vi "Wago DO Arrange.vi"(0 "Wago Data Input in":T2 {"Input Process Image"."Software Constants"."Room PID Settings"."Room Dehumid Temperature I (*RM Dehum I1)" max=30000 step=1; "Input Process Image"."Software Constants"."Room PID Settings"."Room Dehumid Temperature P (*RM Dehum P1)" max=30000 step=1; "Input Process Image"."Software Constants"."Room PID Settings"."Room Cool Temperature I (*RM Cool I1)" max=30000 step=1; "Input Process Image"."Software Constants"."Room PID Settings"."Room Cool Temperature P (*RM Cool P1)" max=30000 step=1; "Input Process Image"."Software Constants"."Room PID Settings"."Room Heat I (*RM Heat I1)" max=30000 step=1; "Input Process Image"."Software Constants"."Room PID Settings"."Room Heat P (*RM Heat P1)" max=30000 step=1; "Input Process Image"."Software Constants"."Room PID Settings"."Room Humidity I (*RM Hum I1)" max=30000 step=1; "Input Process Image"."Software Constants"."Room PID Settings"."Room Humidity P (*RM Hum P1)" max=30000 step=1; "Input Process Image"."Software Constants"."Room PID Settings"."Room Dry I (*RM Dry I1)" max=30000 step=1; "Input Process Image"."Software Constants"."Room PID Settings"."Room Dry P(*RM Dry P1)" max=30000 step=1}, 5 "Flipped Bytes (16 bits)":bool[](array[boolean]), 11 "Error In":errorcluster, 12 "Wago Output Words":T1=519 items=["twHeatCtrl"=512, "twSteamCtrl"=513, "twCoolCtrl"=514, "twDehumCtrl"=515, "Output QX4 Bool"=516, "Output QX5 Bool"=517, "Output QX6 Bool"=518, "Output QX7 Bool"=519, "Output QX8 Bool"=520, "Output QX9 Bool"=521, "Output QX10"=522, "twRoomTemp"=840, "twRoomHum"=841, "twSuppTemp"=842, "twCoolTemp"=843, "twDehumTemp"=844, "twGlycolTemp"=845, "twHeatRate"=846, "twSteamRate"=847, "twCoolRate"=848, "twDehumRate"=849, "twStatus"=850, "twDoorEna"=851, "Rm1St1Dr1Stat"=816, "Rm1St2Dr1Stat"=817, "Rm1St3Dr1Stat"=818, "Rm1St4Dr1Stat"=819, "Rm1St5Dr1Stat"=820, "Rm1St6Dr1Stat"=821, "Rm1St7Dr1Stat"=822, "Rm1St8Dr1Stat"=823, "Rm1St1Dr2Stat"=824, "Rm1St2Dr2Stat"=825, "Rm1St3Dr2Stat"=826, "Rm1St4Dr2Stat"=827, "Rm1St5Dr2Stat"=828, "Rm1St6DrStat"=829, "Rm1St7Dr2Stat"=830, "Rm1St8Dr2Stat"=831, "Rm1St1Dr3Stat"=832, "Rm1St2Dr3Stat"=833, "Rm1St3Dr3Stat"=834, "Rm1St4Dr3Stat"=835, "Rm1St5Dr3Stat"=836, "Rm1St6Dr3Stat"=837, "Rm1St7Dr3Stat"=838, "Rm1St8Dr3Stat"=839, "twVoltMon1"=784, "twVoltMon2"=785, "twVoltMon3"=786, "twVoltMon4"=787, "twVoltMon5"=788, "twVoltMon6"=789, "twVoltMon7"=790, "twVoltMon8"=791, "twVoltStat1"=792, "twVoltStat2"=793, "twVoltStat3"=794, "twVoltStat4"=795, "twVoltStat5"=796, "twVoltStat6"=797, "twVoltStat7"=798, "twVoltStat8"=799]) -> (4 "Wago Data Input out":T2 {"Input Process Image"."Software Constants"."Room PID Settings"."Room Dehumid Temperature I (*RM Dehum I1)" max=30000 step=1; "Input Process Image"."Software Constants"."Room PID Settings"."Room Dehumid Temperature P (*RM Dehum P1)" max=30000 step=1; "Input Process Image"."Software Constants"."Room PID Settings"."Room Cool Temperature I (*RM Cool I1)" max=30000 step=1; "Input Process Image"."Software Constants"."Room PID Settings"."Room Cool Temperature P (*RM Cool P1)" max=30000 step=1; "Input Process Image"."Software Constants"."Room PID Settings"."Room Heat I (*RM Heat I1)" max=30000 step=1; "Input Process Image"."Software Constants"."Room PID Settings"."Room Heat P (*RM Heat P1)" max=30000 step=1; "Input Process Image"."Software Constants"."Room PID Settings"."Room Humidity I (*RM Hum I1)" max=30000 step=1; "Input Process Image"."Software Constants"."Room PID Settings"."Room Humidity P (*RM Hum P1)" max=30000 step=1; "Input Process Image"."Software Constants"."Room PID Settings"."Room Dry I (*RM Dry I1)" max=30000 step=1; "Input Process Image"."Software Constants"."Room PID Settings"."Room Dry P(*RM Dry P1)" max=30000 step=1}, 15 "Error Out":errorcluster)   [LabVIEW 2016]
uses:
  Type Definitions/Wago Main Control.ctl
  Type Definitions/Wago Output Data Process Image.ctl
  Type Definitions/Wago Room Condtions.ctl
  Type Definitions/Wago Door Relays.ctl
  Type Definitions/Wago Contactor Settings.ctl
  Type Definitions/Wago Ground Leakage.ctl
  Type Definitions/Wago Input Process Image.ctl
  Type Definitions/Wago Room PID Settings.ctl
  Type Definitions/Wago Measured Input Data.ctl
  Type Definitions/Wago Room Setpoint Targets.ctl
  Type Definitions/Wago Output Commands.ctl
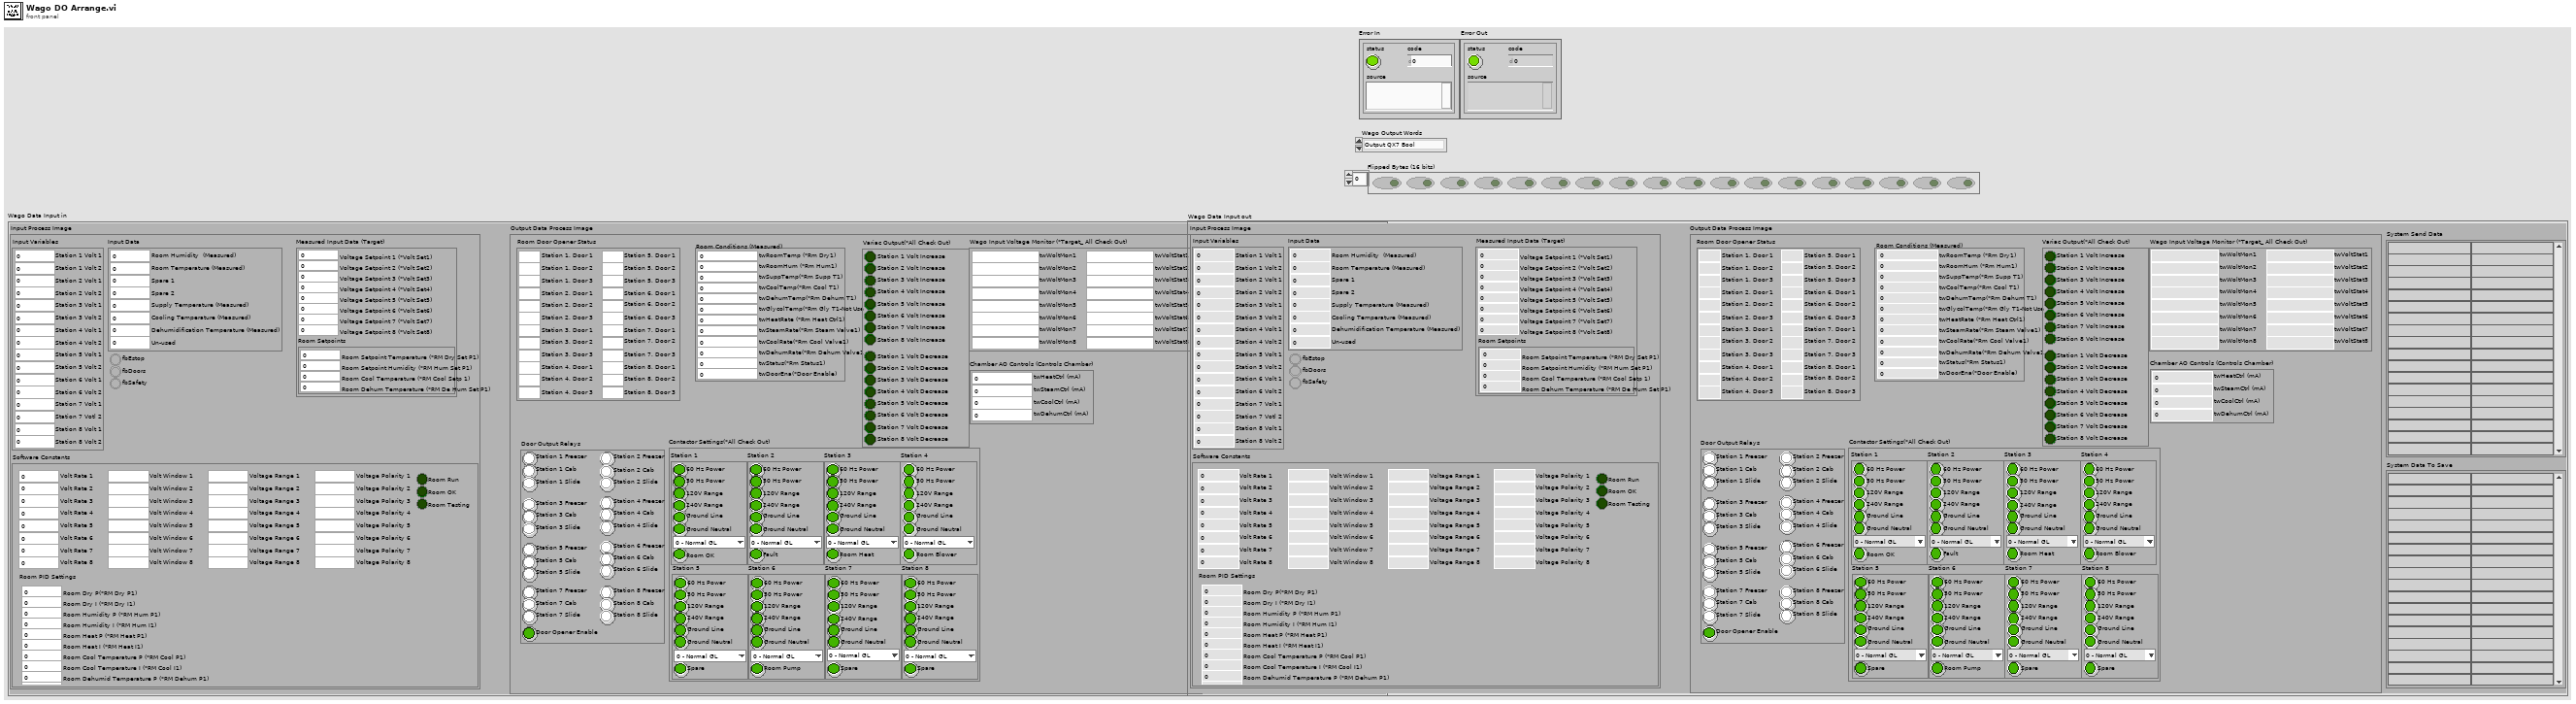
[diagram p1: front panel]
types:
  T1 = typedef "Wago Output Commands.ctl" = u16
  T2 = typedef "Wago Main Control.ctl" = cluster{"Output Data Process Image":T3, "Input Process Image":T8, "System Send Data":string[][], "System Data To Save":string[][]}
  T3 = typedef "Wago Output Data Process Image.ctl" = cluster{"Room Door Opener Status":cluster{"Station 1, Door 1":u16, "Station 1, Door 2":u16, "Station 1, Door 3":u16, "Station 2, Door 1":u16, "Station 2, Door 2":u16, "Station 2, Door 3":u16, "Station 3, Door 1":u16, "Station 3, Door 2":u16, "Station 3, Door 3":u16, "Station 4, Door 1":u16, "Station 4, Door 2":u16, "Station 4, Door 3":u16, "Station 5, Door 1":u16, "Station 5, Door 2":u16, "Station 5, Door 3":u16, "Station 6, Door 1":u16, "Station 6, Door 2":u16, "Station 6, Door 3":u16, "Station 7, Door 1":u16, "Station 7, Door 2":u16, "Station 7, Door 3":u16, "Station 8, Door 1":u16, "Station 8, Door 2":u16, "Station 8, Door 3":u16}, "Room Conditions (Measured)":T4, "Chamber AO Controls (Controls Chamber)":cluster{"twDehumCtrl (mA)":u16, "twCoolCtrl (mA)":u16, "twSteamCtrl (mA)":u16, "twHeatCtrl (mA)":u16}, "Variac Output(*All Check Out)":cluster{"Station 1 Volt Increase":bool, "Station 1 Volt Decrease":bool, "Station 2 Volt Increase":bool, "Station 2 Volt Decrease":bool, "Station 3 Volt Increase":bool, "Station 3 Volt Decrease":bool, "Station 4 Volt Increase":bool, "Station 4 Volt Decrease":bool, "Station 5 Volt Increase":bool, "Station 5 Volt Decrease":bool, "Station 6 Volt Increase":bool, "Station 6 Volt Decrease":bool, "Station 7 Volt Increase":bool, "Station 7 Volt Decrease":bool, "Station 8 Volt Increase":bool, "Station 8 Volt Decrease":bool}, "Door Output Relays":T5, "Wago Input Voltage Monitor (*Target_ All Check Out)":cluster{"twWoltMon1":dbl, "twWoltMon2":dbl, "twWoltMon3":dbl, "twWoltMon4":dbl, "twWoltMon5":dbl, "twWoltMon6":dbl, "twWoltMon7":dbl, "twWoltMon8":dbl, "twVoltStat1":u16, "twVoltStat2":u16, "twVoltStat3":u16, "twVoltStat4":u16, "twVoltStat5":u16, "twVoltStat6":u16, "twVoltStat7":u16, "twVoltStat8":u16}, "Contactor Settings(*All Check Out)":T6}
  T4 = typedef "Wago Room Condtions.ctl" = cluster{"twDoorEna(*Door Enable)":u16, "twStatus(*Rm Status1)":u16, "twRoomTemp (*Rm Dry1)":dbl, "twRoomHum (*Rm Hum1)":dbl, "twSuppTemp(*Rm Supp T1)":dbl, "twCoolTemp(*Rm Cool T1)":dbl, "twDehumTemp(*Rm Dehum T1)":dbl, "twGlycolTemp(*Rm Gly T1-Not Used)":dbl, "twDehumRate(*Rm Dehum Valve1)":dbl, "twCoolRate(*Rm Cool Valve1)":dbl, "twSteamRate(*Rm Steam Valve1)":dbl, "twHeatRate (*Rm Heat Ctrl1)":dbl}
  T5 = typedef "Wago Door Relays.ctl" = cluster{"Station 1 Freezer":bool, "Station 1 Cab":bool, "Station 1 Slide":bool, "Station 2 Freezer":bool, "Station 2 Cab":bool, "Station 2 Slide":bool, "Station 3 Freezer":bool, "Station 3 Cab":bool, "Station 3 Slide":bool, "Station 4 Freezer":bool, "Station 4 Cab":bool, "Station 4 Slide":bool, "Station 5 Freezer":bool, "Station 5 Cab":bool, "Station 5 Slide":bool, "Station 6 Freezer":bool, "Station 6 Cab":bool, "Station 6 Slide":bool, "Station 7 Freezer":bool, "Station 7 Cab":bool, "Station 7 Slide":bool, "Station 8 Freezer":bool, "Station 8 Cab":bool, "Station 8 Slide":bool, "Door Opener Enable":bool}
  T6 = typedef "Wago Contactor Settings.ctl" = cluster{"Station 1":cluster{"60 Hz Power":bool, "50 Hz Power":bool, "120V Range":bool, "240V Range":bool, "Ground Line":bool, "Ground Neutral":bool, "Room OK":bool, "Ground Leakage":T7}, "Station 2":cluster{"60 Hz Power":bool, "50 Hz Power":bool, "120V Range":bool, "240V Range":bool, "Ground Line":bool, "Ground Neutral":bool, "Fault":bool, "Ground Leakage":T7}, "Station 3":cluster{"60 Hz Power":bool, "50 Hz Power":bool, "120V Range":bool, "240V Range":bool, "Ground Line":bool, "Ground Neutral":bool, "Room Heat":bool, "Ground Leakage":T7}, "Station 4":cluster{"60 Hz Power":bool, "50 Hz Power":bool, "120V Range":bool, "240V Range":bool, "Ground Line":bool, "Ground Neutral":bool, "Room Blower":bool, "Ground Leakage":T7}, "Station 5":cluster{"60 Hz Power":bool, "50 Hz Power":bool, "120V Range":bool, "240V Range":bool, "Ground Line":bool, "Ground Neutral":bool, "Spare":bool, "Ground Leakage":T7}, "Station 6":cluster{"60 Hz Power":bool, "50 Hz Power":bool, "120V Range":bool, "240V Range":bool, "Ground Line":bool, "Ground Neutral":bool, "Room Pump":bool, "Ground Leakage":T7}, "Station 7":cluster{"60 Hz Power":bool, "50 Hz Power":bool, "120V Range":bool, "240V Range":bool, "Ground Line":bool, "Ground Neutral":bool, "Spare":bool, "Ground Leakage":T7}, "Station 8":cluster{"60 Hz Power":bool, "50 Hz Power":bool, "120V Range":bool, "240V Range":bool, "Ground Line":bool, "Ground Neutral":bool, "Spare":bool, "Ground Leakage":T7}}
  T7 = typedef "Wago Ground Leakage.ctl" = enum16{"0 - Normal GL", "1 - Measure GL"}
  T8 = typedef "Wago Input Process Image.ctl" = cluster{"fbEstop":bool, "fbDoors":bool, "fbSafety":bool, "Input Variables":cluster{"Station 1 Volt 1":dbl, "Station 1 Volt 2":dbl, "Station 2 Volt 1":dbl, "Station 2 Volt 2":dbl, "Station 3 Volt 1":dbl, "Station 3 Volt 2":dbl, "Station 4 Volt 1":dbl, "Station 4 Volt 2":dbl, "Station 5 Volt 1":dbl, "Station 5 Volt 2":dbl, "Station 6 Volt 1":dbl, "Station 6 Volt 2":dbl, "Station 7 Volt 1":dbl, "Station 7 Votl 2":dbl, "Station 8 Volt 1":dbl, "Station 8 Volt 2":dbl}, "Input Data":cluster{"Room Humidity  (Measured)":dbl, "Room Temperature (Measured)":dbl, "Spare 1":dbl, "Spare 2":dbl, "Supply Temperature (Measured)":dbl, "Cooling Temperature (Measured)":dbl, "Dehumidification Temperature (Measured)":dbl, "Un-used":dbl}, "Software Constants":cluster{"Volt Rate 1":u16, "Volt Rate 2":u16, "Volt Rate 3":u16, "Volt Rate 4":u16, "Volt Rate 5":u16, "Volt Rate 6":u16, "Volt Rate 7":u16, "Volt Rate 8":u16, "Volt Window 1":u16, "Volt Window 2":u16, "Volt Window 3":u16, "Volt Window 4":u16, "Volt Window 5":u16, "Volt Window 6":u16, "Volt Window 7":u16, "Volt Window 8":u16, "Voltage Range 1":u16, "Voltage Range 2":u16, "Voltage Range 3":u16, "Voltage Range 4":u16, "Voltage Range 5":u16, "Voltage Range 6":u16, "Voltage Range 7":u16, "Voltage Range 8":u16, "Voltage Polarity 1":u16, "Voltage Polarity 2":u16, "Voltage Polarity 3":u16, "Voltage Polarity 4":u16, "Voltage Polarity 5":u16, "Voltage Polarity 6":u16, "Voltage Polarity 7":u16, "Voltage Polarity 8":u16, "Room Run":bool, "Room OK":bool, "Room Testing":bool, "Room PID Settings":T9}, "Measured Input Data (Target)":T10}
  T9 = typedef "Wago Room PID Settings.ctl" = cluster{"Room Dry P(*RM Dry P1)":u16, "Room Dry I (*RM Dry I1)":u16, "Room Humidity P (*RM Hum P1)":u16, "Room Humidity I (*RM Hum I1)":u16, "Room Heat P (*RM Heat P1)":u16, "Room Heat I (*RM Heat I1)":u16, "Room Cool Temperature P (*RM Cool P1)":u16, "Room Cool Temperature I (*RM Cool I1)":u16, "Room Dehumid Temperature P (*RM Dehum P1)":u16, "Room Dehumid Temperature I (*RM Dehum I1)":u16}
  T10 = typedef "Wago Measured Input Data.ctl" = cluster{"Voltage Setpoint 1 (*Volt Set1)":dbl, "Voltage Setpoint 2 (*Volt Set2)":dbl, "Voltage Setpoint 3 (*Volt Set3)":dbl, "Voltage Setpoint 4 (*Volt Set4)":dbl, "Voltage Setpoint 5 (*Volt Set5)":dbl, "Voltage Setpoint 6 (*Volt Set6)":dbl, "Voltage Setpoint 7 (*Volt Set7)":dbl, "Voltage Setpoint 8 (*Volt Set8)":dbl, "Room Setpoints":T11}
  T11 = typedef "Wago Room Setpoint Targets.ctl" = cluster{"Room Setpoint Temperature (*RM Dry Set P1)":dbl, "Room Setpoint Humidity (*RM Hum Set P1)":dbl, "Room Cool Temperature (*RM Cool Setp 1)":dbl, "Room Dehum Temperature (*RM De Hum Set P1)":dbl}
  T12 = cluster{"60 Hz Power":bool, "50 Hz Power":bool, "120V Range":bool, "240V Range":bool, "Ground Line":bool, "Ground Neutral":bool, "Room OK":bool, "Ground Leakage":T7}
  T13 = cluster{"60 Hz Power":bool, "50 Hz Power":bool, "120V Range":bool, "240V Range":bool, "Ground Line":bool, "Ground Neutral":bool, "Fault":bool, "Ground Leakage":T7}
  T14 = cluster{"60 Hz Power":bool, "50 Hz Power":bool, "120V Range":bool, "240V Range":bool, "Ground Line":bool, "Ground Neutral":bool, "Room Heat":bool, "Ground Leakage":T7}
  T15 = cluster{"60 Hz Power":bool, "50 Hz Power":bool, "120V Range":bool, "240V Range":bool, "Ground Line":bool, "Ground Neutral":bool, "Room Blower":bool, "Ground Leakage":T7}
  T16 = cluster{"60 Hz Power":bool, "50 Hz Power":bool, "120V Range":bool, "240V Range":bool, "Ground Line":bool, "Ground Neutral":bool, "Spare":bool, "Ground Leakage":T7}
  T17 = cluster{"60 Hz Power":bool, "50 Hz Power":bool, "120V Range":bool, "240V Range":bool, "Ground Line":bool, "Ground Neutral":bool, "Room Pump":bool, "Ground Leakage":T7}
  T18 = cluster{"Station 1 Volt Increase":bool, "Station 1 Volt Decrease":bool, "Station 2 Volt Increase":bool, "Station 2 Volt Decrease":bool, "Station 3 Volt Increase":bool, "Station 3 Volt Decrease":bool, "Station 4 Volt Increase":bool, "Station 4 Volt Decrease":bool, "Station 5 Volt Increase":bool, "Station 5 Volt Decrease":bool, "Station 6 Volt Increase":bool, "Station 6 Volt Decrease":bool, "Station 7 Volt Increase":bool, "Station 7 Volt Decrease":bool, "Station 8 Volt Increase":bool, "Station 8 Volt Decrease":bool}
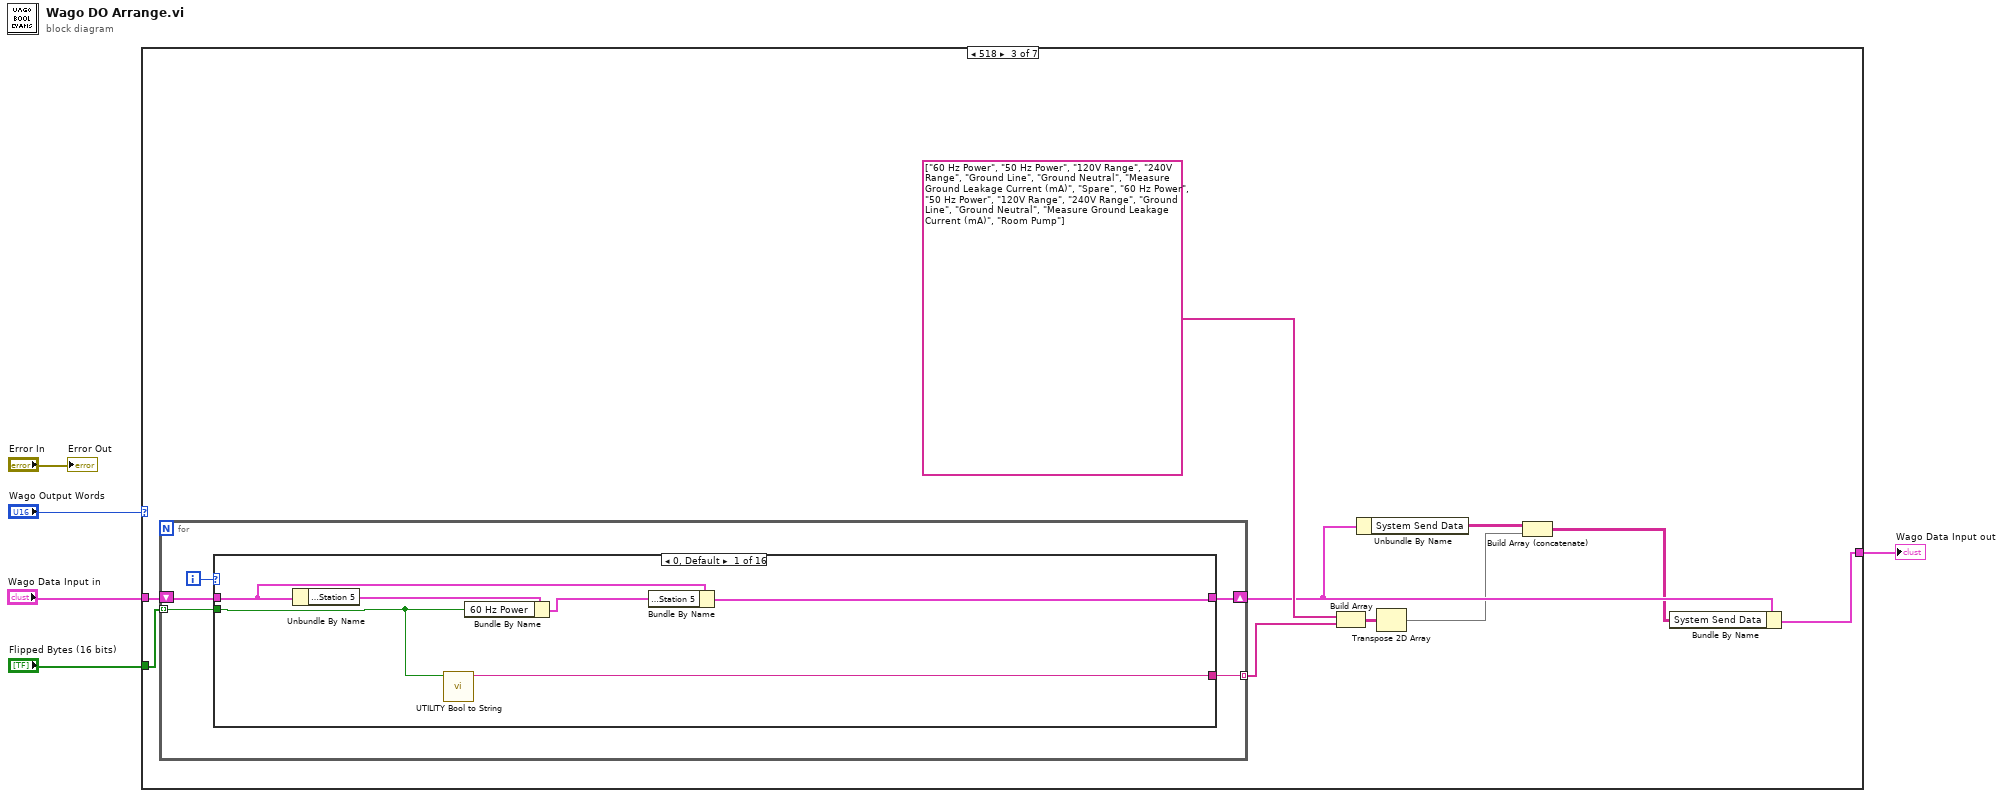
[diagram p0: block diagram]
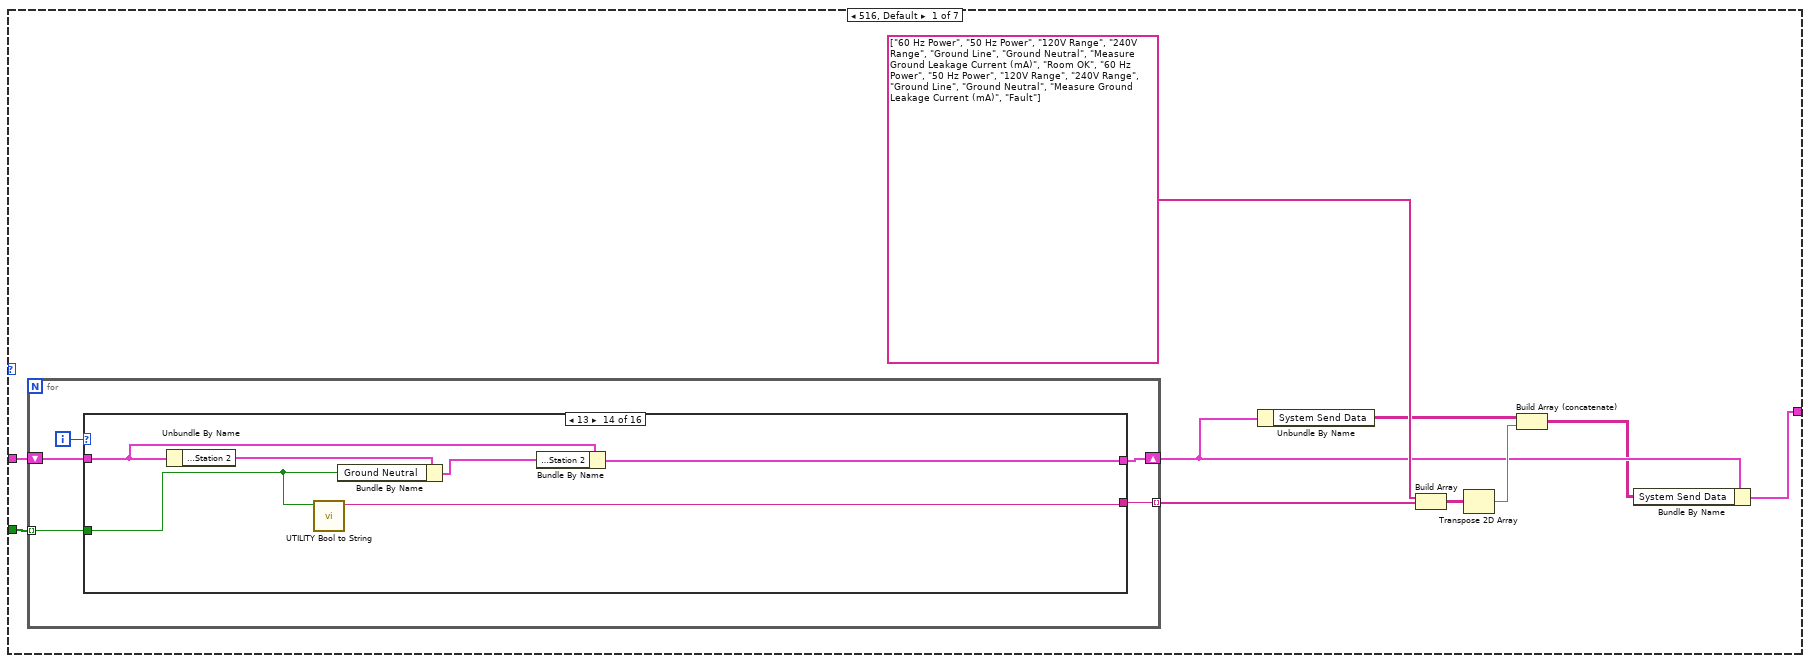
[diagram p2: hidden frame]
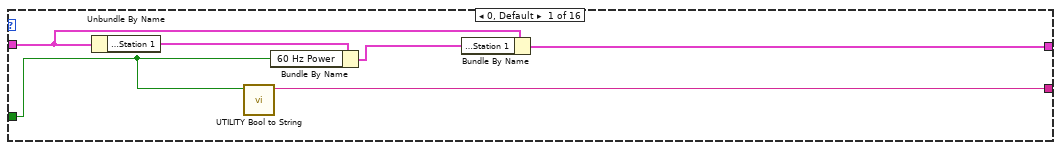
[diagram p3: hidden frame]
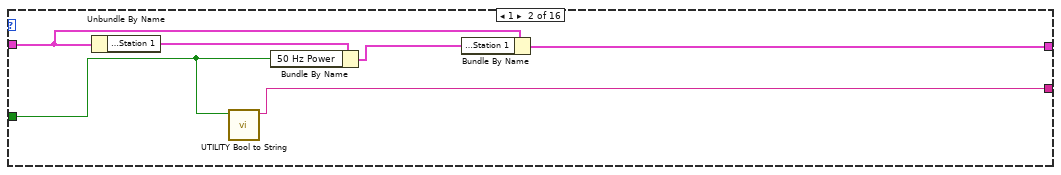
[diagram p4: hidden frame]
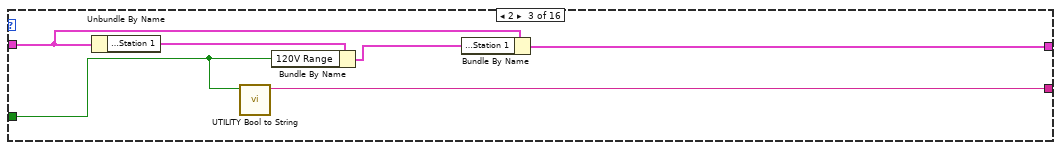
[diagram p5: hidden frame]
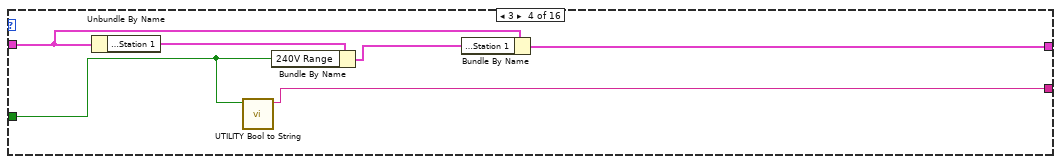
[diagram p6: hidden frame]
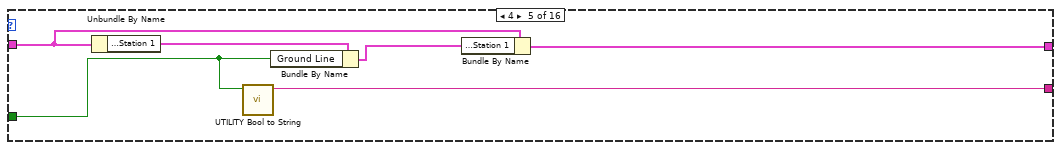
[diagram p7: hidden frame]
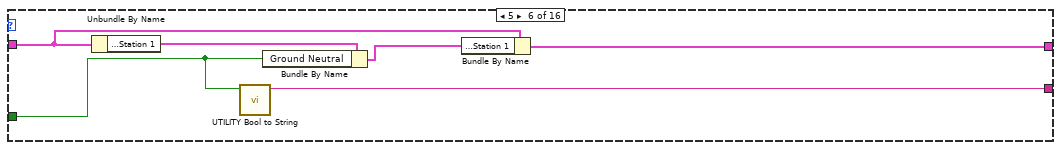
[diagram p8: hidden frame]
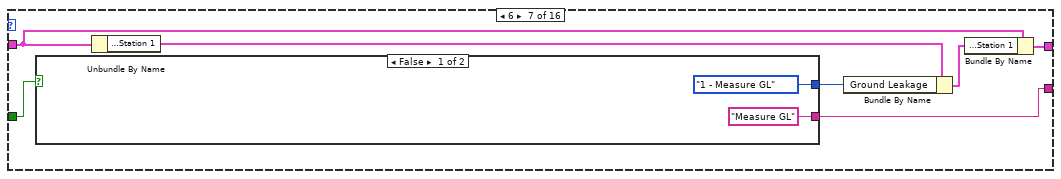
[diagram p9: hidden frame]
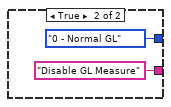
[diagram p10: hidden frame]
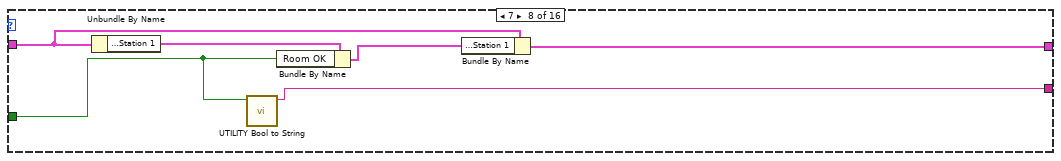
[diagram p11: hidden frame]
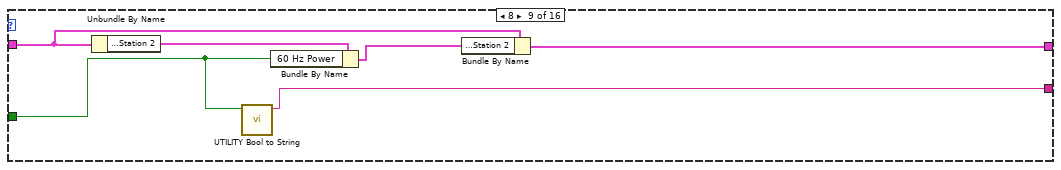
[diagram p12: hidden frame]
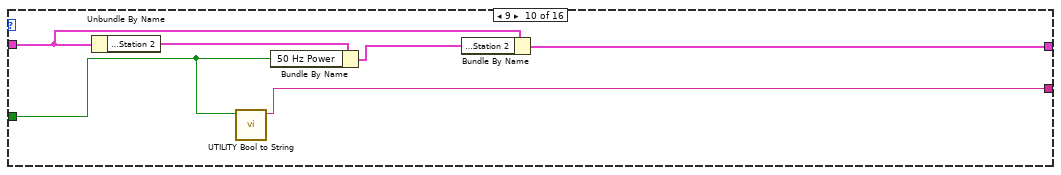
[diagram p13: hidden frame]
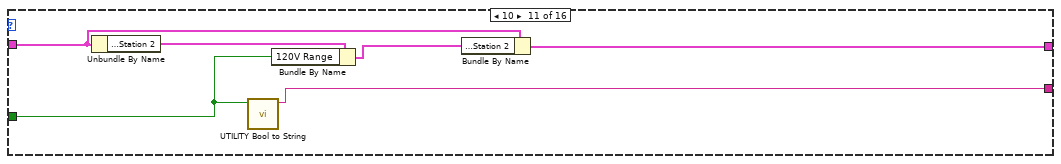
[diagram p14: hidden frame]
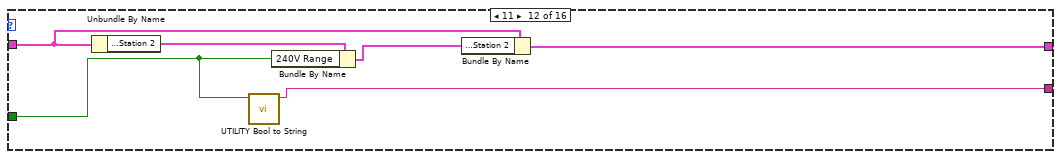
[diagram p15: hidden frame]
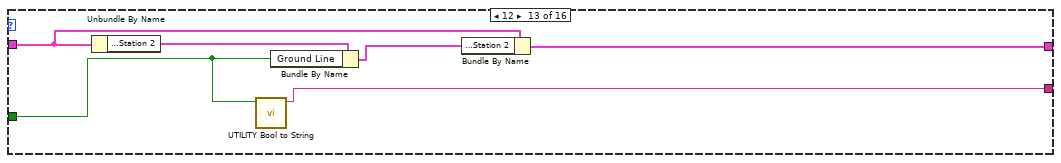
[diagram p16: hidden frame]
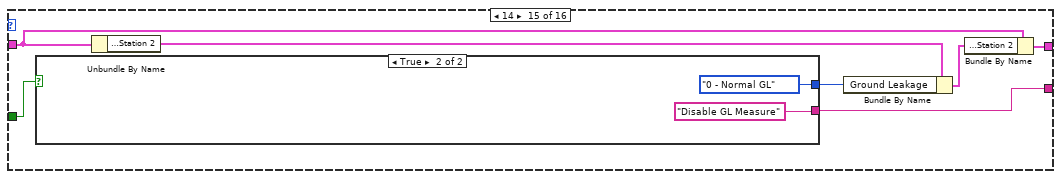
[diagram p17: hidden frame]
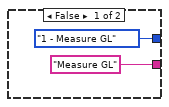
[diagram p18: hidden frame]
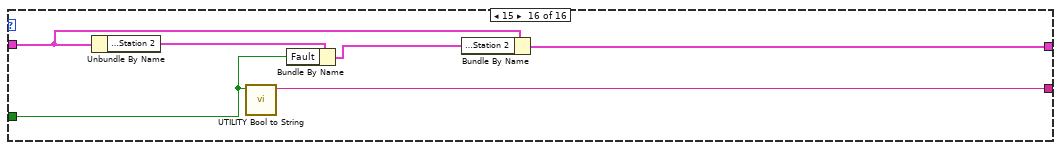
[diagram p19: hidden frame]
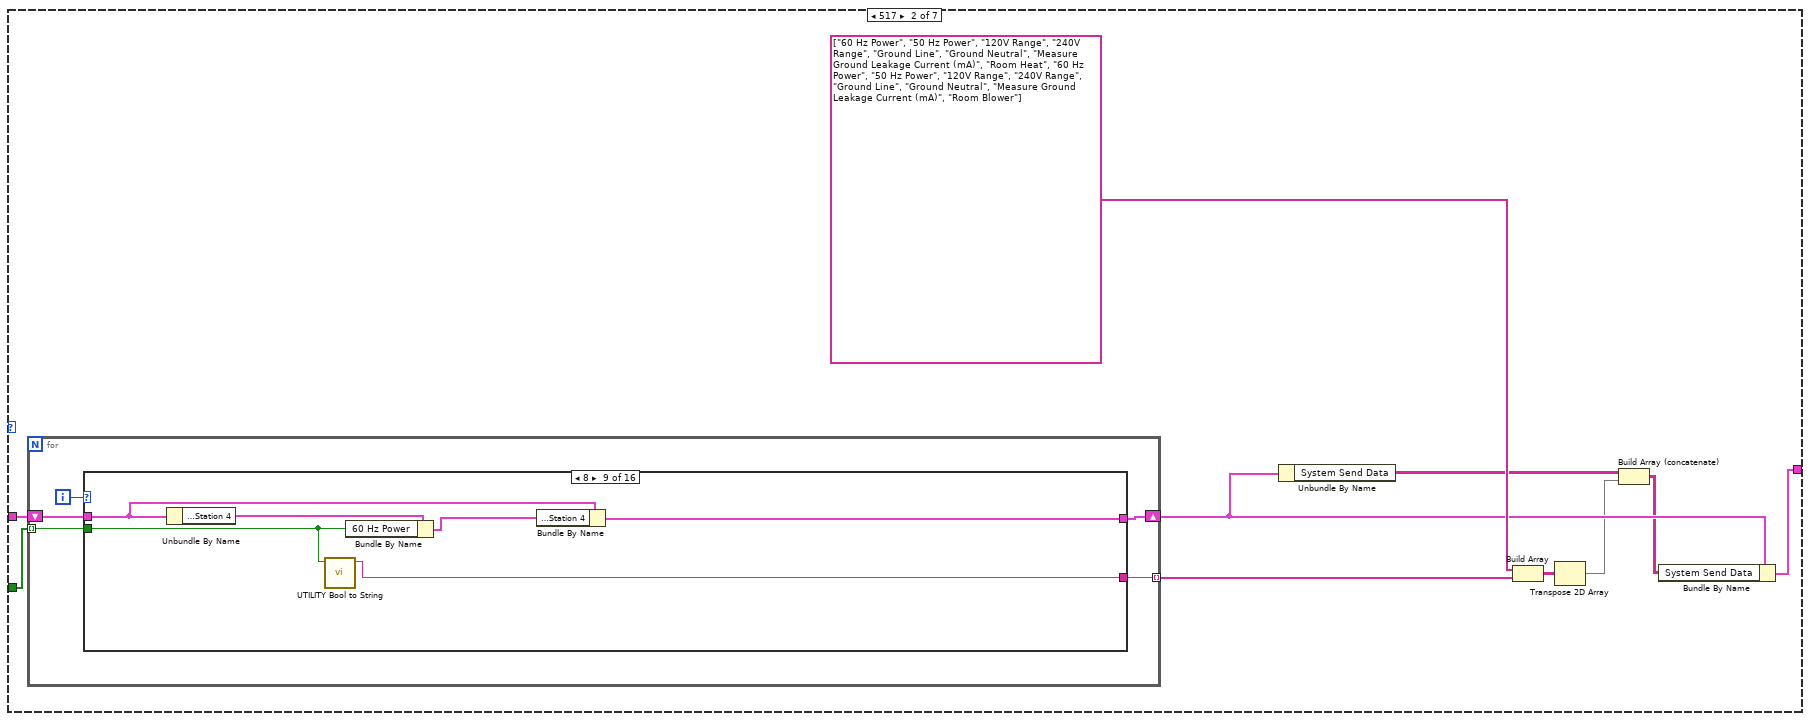
[diagram p20: hidden frame]
diagram:
  n1 = case shown="518" "Wago Output Words" {
    tunnel: "Wago Data Input in" -> [w15 w136 w257 w378 w499 w610 w722]
    tunnel: "Flipped Bytes (16 bits)" -> [w14 w135 w256 w377 w498 w609 w721]
    tunnel: [w10 w131 w254 w375 w496 w607 w718] -> w3
    frame 516, Default {
      n2 = for {
        tunnel: w14 -> [w18] mode=indexing
        shift-right: [w17] -> w8
        shift-left: w15 -> [w20]
        tunnel: [w16] -> w12 mode=indexing
        i -> [w19]
        n3 = case shown="13" w19 {
          tunnel: w20 -> [w25 w30 w36 w42 w48 w54 w61 w71 w77 w83 w89 w95 w101 w107 w114 w124]
          tunnel: w18 -> [w22 w28 w34 w40 w46 w52 w59 w69 w75 w81 w87 w93 w99 w105 w112 w122]
          tunnel: [w23 w29 w35 w41 w47 w53 w60 w70 w76 w82 w88 w94 w100 w106 w113 w123] -> w17
          tunnel: [w21 w27 w33 w39 w45 w51 w57 w68 w74 w80 w86 w92 w98 w104 w110 w121] -> w16
          frame 0, Default {
            n4 = Unbundle By Name(w25) -> ("Output Data Process Image.Contactor Settings(*All Check Out).Station 1"=w26:T12)
            n5 = call "UTILITY Bool to String.vi"("Input Bool"=w22) -> ("Output String"=w21:string)  [unwired: 10 in]
            n6 = Bundle By Name(cluster=w26, "60 Hz Power"=w22) -> (w24:T12)
            n7 = Bundle By Name(cluster=w25, "Output Data Process Image.Contactor Settings(*All Check Out).Station 1"=w24) -> (w23:T2)
          }
          frame 1 {
            n8 = Unbundle By Name(w30) -> ("Output Data Process Image.Contactor Settings(*All Check Out).Station 1"=w32:T12)
            n9 = call "UTILITY Bool to String.vi"("Input Bool"=w28) -> ("Output String"=w27:string)  [unwired: 10 in]
            n10 = Bundle By Name(cluster=w32, "50 Hz Power"=w28) -> (w31:T12)
            n11 = Bundle By Name(cluster=w30, "Output Data Process Image.Contactor Settings(*All Check Out).Station 1"=w31) -> (w29:T2)
          }
          frame 2 {
            n12 = Unbundle By Name(w36) -> ("Output Data Process Image.Contactor Settings(*All Check Out).Station 1"=w38:T12)
            n13 = call "UTILITY Bool to String.vi"("Input Bool"=w34) -> ("Output String"=w33:string)  [unwired: 10 in]
            n14 = Bundle By Name(cluster=w38, "120V Range"=w34) -> (w37:T12)
            n15 = Bundle By Name(cluster=w36, "Output Data Process Image.Contactor Settings(*All Check Out).Station 1"=w37) -> (w35:T2)
          }
          frame 3 {
            n16 = Unbundle By Name(w42) -> ("Output Data Process Image.Contactor Settings(*All Check Out).Station 1"=w44:T12)
            n17 = call "UTILITY Bool to String.vi"("Input Bool"=w40) -> ("Output String"=w39:string)  [unwired: 10 in]
            n18 = Bundle By Name(cluster=w44, "240V Range"=w40) -> (w43:T12)
            n19 = Bundle By Name(cluster=w42, "Output Data Process Image.Contactor Settings(*All Check Out).Station 1"=w43) -> (w41:T2)
          }
          frame 4 {
            n20 = Unbundle By Name(w48) -> ("Output Data Process Image.Contactor Settings(*All Check Out).Station 1"=w50:T12)
            n21 = call "UTILITY Bool to String.vi"("Input Bool"=w46) -> ("Output String"=w45:string)  [unwired: 10 in]
            n22 = Bundle By Name(cluster=w50, "Ground Line"=w46) -> (w49:T12)
            n23 = Bundle By Name(cluster=w48, "Output Data Process Image.Contactor Settings(*All Check Out).Station 1"=w49) -> (w47:T2)
          }
          frame 5 {
            n24 = Unbundle By Name(w54) -> ("Output Data Process Image.Contactor Settings(*All Check Out).Station 1"=w56:T12)
            n25 = call "UTILITY Bool to String.vi"("Input Bool"=w52) -> ("Output String"=w51:string)  [unwired: 10 in]
            n26 = Bundle By Name(cluster=w56, "Ground Neutral"=w52) -> (w55:T12)
            n27 = Bundle By Name(cluster=w54, "Output Data Process Image.Contactor Settings(*All Check Out).Station 1"=w55) -> (w53:T2)
          }
          frame 6 {
            n28 = case shown="False" w59 {
              tunnel: [Wago_Ground_Leakage."1 - Measure GL" ("Ground Leakage") Wago_Ground_Leakage."0 - Normal GL" ("Ground Leakage")] -> w58
              tunnel: ["Measure GL" "Disable GL Measure"] -> w57
              frame False {
              }
              frame True {
              }
            }
            n29 = Unbundle By Name(w61) -> ("Output Data Process Image.Contactor Settings(*All Check Out).Station 1"=w63:T12)
            n30 = Bundle By Name(cluster=w63, "Ground Leakage"=w58) -> (w62:T12)
            n31 = Bundle By Name(cluster=w61, "Output Data Process Image.Contactor Settings(*All Check Out).Station 1"=w62) -> (w60:T2)
          }
          frame 7 {
            n32 = Unbundle By Name(w71) -> ("Output Data Process Image.Contactor Settings(*All Check Out).Station 1"=w73:T12)
            n33 = call "UTILITY Bool to String.vi"("Input Bool"=w69) -> ("Output String"=w68:string)  [unwired: 10 in]
            n34 = Bundle By Name(cluster=w73, "Room OK"=w69) -> (w72:T12)
            n35 = Bundle By Name(cluster=w71, "Output Data Process Image.Contactor Settings(*All Check Out).Station 1"=w72) -> (w70:T2)
          }
          frame 8 {
            n36 = Unbundle By Name(w77) -> ("Output Data Process Image.Contactor Settings(*All Check Out).Station 2"=w79:T13)
            n37 = call "UTILITY Bool to String.vi"("Input Bool"=w75) -> ("Output String"=w74:string)  [unwired: 10 in]
            n38 = Bundle By Name(cluster=w79, "60 Hz Power"=w75) -> (w78:T13)
            n39 = Bundle By Name(cluster=w77, "Output Data Process Image.Contactor Settings(*All Check Out).Station 2"=w78) -> (w76:T2)
          }
          frame 9 {
            n40 = Unbundle By Name(w83) -> ("Output Data Process Image.Contactor Settings(*All Check Out).Station 2"=w85:T13)
            n41 = call "UTILITY Bool to String.vi"("Input Bool"=w81) -> ("Output String"=w80:string)  [unwired: 10 in]
            n42 = Bundle By Name(cluster=w85, "50 Hz Power"=w81) -> (w84:T13)
            n43 = Bundle By Name(cluster=w83, "Output Data Process Image.Contactor Settings(*All Check Out).Station 2"=w84) -> (w82:T2)
          }
          frame 10 {
            n44 = Unbundle By Name(w89) -> ("Output Data Process Image.Contactor Settings(*All Check Out).Station 2"=w91:T13)
            n45 = call "UTILITY Bool to String.vi"("Input Bool"=w87) -> ("Output String"=w86:string)  [unwired: 10 in]
            n46 = Bundle By Name(cluster=w91, "120V Range"=w87) -> (w90:T13)
            n47 = Bundle By Name(cluster=w89, "Output Data Process Image.Contactor Settings(*All Check Out).Station 2"=w90) -> (w88:T2)
          }
          frame 11 {
            n48 = Unbundle By Name(w95) -> ("Output Data Process Image.Contactor Settings(*All Check Out).Station 2"=w97:T13)
            n49 = call "UTILITY Bool to String.vi"("Input Bool"=w93) -> ("Output String"=w92:string)  [unwired: 10 in]
            n50 = Bundle By Name(cluster=w97, "240V Range"=w93) -> (w96:T13)
            n51 = Bundle By Name(cluster=w95, "Output Data Process Image.Contactor Settings(*All Check Out).Station 2"=w96) -> (w94:T2)
          }
          frame 12 {
            n52 = Unbundle By Name(w101) -> ("Output Data Process Image.Contactor Settings(*All Check Out).Station 2"=w103:T13)
            n53 = call "UTILITY Bool to String.vi"("Input Bool"=w99) -> ("Output String"=w98:string)  [unwired: 10 in]
            n54 = Bundle By Name(cluster=w103, "Ground Line"=w99) -> (w102:T13)
            n55 = Bundle By Name(cluster=w101, "Output Data Process Image.Contactor Settings(*All Check Out).Station 2"=w102) -> (w100:T2)
          }
          frame 13 {
            n56 = Unbundle By Name(w107) -> ("Output Data Process Image.Contactor Settings(*All Check Out).Station 2"=w109:T13)
            n57 = call "UTILITY Bool to String.vi"("Input Bool"=w105) -> ("Output String"=w104:string)  [unwired: 10 in]
            n58 = Bundle By Name(cluster=w109, "Ground Neutral"=w105) -> (w108:T13)
            n59 = Bundle By Name(cluster=w107, "Output Data Process Image.Contactor Settings(*All Check Out).Station 2"=w108) -> (w106:T2)
          }
          frame 14 {
            n60 = case shown="True" w112 {
              tunnel: [Wago_Ground_Leakage."1 - Measure GL" ("Ground Leakage") Wago_Ground_Leakage."0 - Normal GL" ("Ground Leakage")] -> w111
              tunnel: ["Measure GL" "Disable GL Measure"] -> w110
              frame False {
              }
              frame True {
              }
            }
            n61 = Unbundle By Name(w114) -> ("Output Data Process Image.Contactor Settings(*All Check Out).Station 2"=w116:T13)
            n62 = Bundle By Name(cluster=w116, "Ground Leakage"=w111) -> (w115:T13)
            n63 = Bundle By Name(cluster=w114, "Output Data Process Image.Contactor Settings(*All Check Out).Station 2"=w115) -> (w113:T2)
          }
          frame 15 {
            n64 = Unbundle By Name(w124) -> ("Output Data Process Image.Contactor Settings(*All Check Out).Station 2"=w126:T13)
            n65 = call "UTILITY Bool to String.vi"("Input Bool"=w122) -> ("Output String"=w121:string)  [unwired: 10 in]
            n66 = Bundle By Name(cluster=w126, "Fault"=w122) -> (w125:T13)
            n67 = Bundle By Name(cluster=w124, "Output Data Process Image.Contactor Settings(*All Check Out).Station 2"=w125) -> (w123:T2)
          }
        }
      }
      n68 = Unbundle By Name(w8) -> ("System Send Data"=w7:string[][])
      n69 = Build Array(string[] ["60 Hz Power", "50 Hz Power", "120V Range", "240V Range", "Ground Line", "Ground Neutral", "Measure Ground Leakage Current (mA)", "Room OK", "60 Hz Power", "50 Hz Power", "120V Range", "240V Range", "Ground Line", "Ground Neutral", "Measure Ground Leakage Current (mA)", "Fault"], w12) -> (w11:string[][])
      n70 = Transpose 2D Array(2D array=w11) -> (transposed array=w9:string[][])
      n71 = Build Array (concatenate)(w7, w9) -> (w6:string[][])
      n72 = Bundle By Name(cluster=w8, "System Send Data"=w6) -> (w10:T2)
    }
    frame 517 {
      n73 = for {
        tunnel: w135 -> [w139] mode=indexing
        shift-right: [w138] -> w129
        shift-left: w136 -> [w141]
        tunnel: [w137] -> w132 mode=indexing
        i -> [w140]
        n74 = case shown="8" w140 {
          tunnel: w141 -> [w146 w151 w157 w163 w169 w175 w182 w192 w198 w204 w210 w216 w222 w228 w235 w245]
          tunnel: w139 -> [w143 w149 w155 w161 w167 w173 w180 w190 w196 w202 w208 w214 w220 w226 w232 w243]
          tunnel: [w144 w150 w156 w162 w168 w174 w181 w191 w197 w203 w209 w215 w221 w227 w234 w244] -> w138
          tunnel: [w142 w148 w154 w160 w166 w172 w178 w189 w195 w201 w207 w213 w219 w225 w231 w242] -> w137
          frame 0, Default {
            n75 = Unbundle By Name(w146) -> ("Output Data Process Image.Contactor Settings(*All Check Out).Station 3"=w147:T14)
            n76 = call "UTILITY Bool to String.vi"("Input Bool"=w143) -> ("Output String"=w142:string)  [unwired: 10 in]
            n77 = Bundle By Name(cluster=w147, "60 Hz Power"=w143) -> (w145:T14)
            n78 = Bundle By Name(cluster=w146, "Output Data Process Image.Contactor Settings(*All Check Out).Station 3"=w145) -> (w144:T2)
          }
          frame 1 {
            n79 = Unbundle By Name(w151) -> ("Output Data Process Image.Contactor Settings(*All Check Out).Station 3"=w153:T14)
            n80 = call "UTILITY Bool to String.vi"("Input Bool"=w149) -> ("Output String"=w148:string)  [unwired: 10 in]
            n81 = Bundle By Name(cluster=w153, "50 Hz Power"=w149) -> (w152:T14)
            n82 = Bundle By Name(cluster=w151, "Output Data Process Image.Contactor Settings(*All Check Out).Station 3"=w152) -> (w150:T2)
          }
          frame 2 {
            n83 = Unbundle By Name(w157) -> ("Output Data Process Image.Contactor Settings(*All Check Out).Station 3"=w159:T14)
            n84 = call "UTILITY Bool to String.vi"("Input Bool"=w155) -> ("Output String"=w154:string)  [unwired: 10 in]
            n85 = Bundle By Name(cluster=w159, "120V Range"=w155) -> (w158:T14)
            n86 = Bundle By Name(cluster=w157, "Output Data Process Image.Contactor Settings(*All Check Out).Station 3"=w158) -> (w156:T2)
          }
          frame 3 {
            n87 = Unbundle By Name(w163) -> ("Output Data Process Image.Contactor Settings(*All Check Out).Station 3"=w165:T14)
            n88 = call "UTILITY Bool to String.vi"("Input Bool"=w161) -> ("Output String"=w160:string)  [unwired: 10 in]
            n89 = Bundle By Name(cluster=w165, "240V Range"=w161) -> (w164:T14)
            n90 = Bundle By Name(cluster=w163, "Output Data Process Image.Contactor Settings(*All Check Out).Station 3"=w164) -> (w162:T2)
          }
          frame 4 {
            n91 = Unbundle By Name(w169) -> ("Output Data Process Image.Contactor Settings(*All Check Out).Station 3"=w171:T14)
            n92 = call "UTILITY Bool to String.vi"("Input Bool"=w167) -> ("Output String"=w166:string)  [unwired: 10 in]
            n93 = Bundle By Name(cluster=w171, "Ground Line"=w167) -> (w170:T14)
            n94 = Bundle By Name(cluster=w169, "Output Data Process Image.Contactor Settings(*All Check Out).Station 3"=w170) -> (w168:T2)
          }
          frame 5 {
            n95 = Unbundle By Name(w175) -> ("Output Data Process Image.Contactor Settings(*All Check Out).Station 3"=w177:T14)
            n96 = call "UTILITY Bool to String.vi"("Input Bool"=w173) -> ("Output String"=w172:string)  [unwired: 10 in]
            n97 = Bundle By Name(cluster=w177, "Ground Neutral"=w173) -> (w176:T14)
            n98 = Bundle By Name(cluster=w175, "Output Data Process Image.Contactor Settings(*All Check Out).Station 3"=w176) -> (w174:T2)
          }
          frame 6 {
            n99 = case shown="False" w180 {
              tunnel: [Wago_Ground_Leakage."1 - Measure GL" ("Ground Leakage") Wago_Ground_Leakage."0 - Normal GL" ("Ground Leakage")] -> w179
              tunnel: ["Measure GL" "Disable GL Measure"] -> w178
              frame False {
              }
              frame True {
              }
            }
            n100 = Unbundle By Name(w182) -> ("Output Data Process Image.Contactor Settings(*All Check Out).Station 3"=w184:T14)
            n101 = Bundle By Name(cluster=w184, "Ground Leakage"=w179) -> (w183:T14)
            n102 = Bundle By Name(cluster=w182, "Output Data Process Image.Contactor Settings(*All Check Out).Station 3"=w183) -> (w181:T2)
          }
          frame 7 {
            n103 = Unbundle By Name(w192) -> ("Output Data Process Image.Contactor Settings(*All Check Out).Station 3"=w194:T14)
            n104 = Bundle By Name(cluster=w194, "Room Heat"=w190) -> (w193:T14)
            n105 = call "UTILITY Bool to String.vi"("Input Bool"=w190) -> ("Output String"=w189:string)  [unwired: 10 in]
            n106 = Bundle By Name(cluster=w192, "Output Data Process Image.Contactor Settings(*All Check Out).Station 3"=w193) -> (w191:T2)
          }
          frame 8 {
            n107 = Unbundle By Name(w198) -> ("Output Data Process Image.Contactor Settings(*All Check Out).Station 4"=w200:T15)
            n108 = call "UTILITY Bool to String.vi"("Input Bool"=w196) -> ("Output String"=w195:string)  [unwired: 10 in]
            n109 = Bundle By Name(cluster=w200, "60 Hz Power"=w196) -> (w199:T15)
            n110 = Bundle By Name(cluster=w198, "Output Data Process Image.Contactor Settings(*All Check Out).Station 4"=w199) -> (w197:T2)
          }
          frame 9 {
            n111 = Unbundle By Name(w204) -> ("Output Data Process Image.Contactor Settings(*All Check Out).Station 4"=w206:T15)
            n112 = call "UTILITY Bool to String.vi"("Input Bool"=w202) -> ("Output String"=w201:string)  [unwired: 10 in]
            n113 = Bundle By Name(cluster=w206, "50 Hz Power"=w202) -> (w205:T15)
            n114 = Bundle By Name(cluster=w204, "Output Data Process Image.Contactor Settings(*All Check Out).Station 4"=w205) -> (w203:T2)
          }
          frame 10 {
            n115 = Unbundle By Name(w210) -> ("Output Data Process Image.Contactor Settings(*All Check Out).Station 4"=w212:T15)
            n116 = call "UTILITY Bool to String.vi"("Input Bool"=w208) -> ("Output String"=w207:string)  [unwired: 10 in]
            n117 = Bundle By Name(cluster=w212, "120V Range"=w208) -> (w211:T15)
            n118 = Bundle By Name(cluster=w210, "Output Data Process Image.Contactor Settings(*All Check Out).Station 4"=w211) -> (w209:T2)
          }
          frame 11 {
            n119 = Unbundle By Name(w216) -> ("Output Data Process Image.Contactor Settings(*All Check Out).Station 4"=w218:T15)
            n120 = call "UTILITY Bool to String.vi"("Input Bool"=w214) -> ("Output String"=w213:string)  [unwired: 10 in]
            n121 = Bundle By Name(cluster=w218, "240V Range"=w214) -> (w217:T15)
            n122 = Bundle By Name(cluster=w216, "Output Data Process Image.Contactor Settings(*All Check Out).Station 4"=w217) -> (w215:T2)
          }
          frame 12 {
            n123 = Unbundle By Name(w222) -> ("Output Data Process Image.Contactor Settings(*All Check Out).Station 4"=w224:T15)
            n124 = call "UTILITY Bool to String.vi"("Input Bool"=w220) -> ("Output String"=w219:string)  [unwired: 10 in]
            n125 = Bundle By Name(cluster=w224, "Ground Line"=w220) -> (w223:T15)
            n126 = Bundle By Name(cluster=w222, "Output Data Process Image.Contactor Settings(*All Check Out).Station 4"=w223) -> (w221:T2)
          }
          frame 13 {
            n127 = Unbundle By Name(w228) -> ("Output Data Process Image.Contactor Settings(*All Check Out).Station 4"=w230:T15)
            n128 = call "UTILITY Bool to String.vi"("Input Bool"=w226) -> ("Output String"=w225:string)  [unwired: 10 in]
            n129 = Bundle By Name(cluster=w230, "Ground Neutral"=w226) -> (w229:T15)
            n130 = Bundle By Name(cluster=w228, "Output Data Process Image.Contactor Settings(*All Check Out).Station 4"=w229) -> (w227:T2)
          }
          frame 14 {
            n131 = case shown="True" w232 {
              tunnel: [Wago_Ground_Leakage."1 - Measure GL" ("Ground Leakage") Wago_Ground_Leakage."0 - Normal GL" ("Ground Leakage")] -> w233
              tunnel: ["Measure GL" "Disable GL Measure"] -> w231
              frame False {
              }
              frame True {
              }
            }
            n132 = Unbundle By Name(w235) -> ("Output Data Process Image.Contactor Settings(*All Check Out).Station 4"=w237:T15)
            n133 = Bundle By Name(cluster=w237, "Ground Leakage"=w233) -> (w236:T15)
            n134 = Bundle By Name(cluster=w235, "Output Data Process Image.Contactor Settings(*All Check Out).Station 4"=w236) -> (w234:T2)
          }
          frame 15 {
            n135 = Unbundle By Name(w245) -> ("Output Data Process Image.Contactor Settings(*All Check Out).Station 4"=w247:T15)
            n136 = Bundle By Name(cluster=w247, "Room Blower"=w243) -> (w246:T15)
            n137 = call "UTILITY Bool to String.vi"("Input Bool"=w243) -> ("Output String"=w242:string)  [unwired: 10 in]
            n138 = Bundle By Name(cluster=w245, "Output Data Process Image.Contactor Settings(*All Check Out).Station 4"=w246) -> (w244:T2)
          }
        }
      }
      n139 = Unbundle By Name(w129) -> ("System Send Data"=w130:string[][])
      n140 = Build Array(string[] ["60 Hz Power", "50 Hz Power", "120V Range", "240V Range", "Ground Line", "Ground Neutral", "Measure Ground Leakage Current (mA)", "Room Heat", "60 Hz Power", "50 Hz Power", "120V Range", "240V Range", "Ground Line", "Ground Neutral", "Measure Ground Leakage Current (mA)", "Room Blower"], w132) -> (w134:string[][])
      n141 = Transpose 2D Array(2D array=w134) -> (transposed array=w128:string[][])
      n142 = Build Array (concatenate)(w130, w128) -> (w127:string[][])
      n143 = Bundle By Name(cluster=w129, "System Send Data"=w127) -> (w131:T2)
    }
    frame 518 {
      n144 = for {
        tunnel: w256 -> [w260] mode=indexing
        shift-right: [w259] -> w251
        shift-left: w257 -> [w262]
        tunnel: [w258] -> w252 mode=indexing
        i -> [w261]
        n145 = case shown="0, Default" w261 {
          tunnel: w262 -> [w267 w272 w278 w284 w290 w296 w303 w313 w319 w325 w331 w337 w343 w349 w356 w366]
          tunnel: w260 -> [w264 w270 w276 w282 w288 w294 w301 w311 w317 w323 w329 w335 w341 w347 w354 w364]
          tunnel: [w265 w271 w277 w283 w289 w295 w302 w312 w318 w324 w330 w336 w342 w348 w355 w365] -> w259
          tunnel: [w263 w269 w275 w281 w287 w293 w299 w310 w316 w322 w328 w334 w340 w346 w352 w363] -> w258
          frame 0, Default {
            n146 = Unbundle By Name(w267) -> ("Output Data Process Image.Contactor Settings(*All Check Out).Station 5"=w268:T16)
            n147 = call "UTILITY Bool to String.vi"("Input Bool"=w264) -> ("Output String"=w263:string)  [unwired: 10 in]
            n148 = Bundle By Name(cluster=w268, "60 Hz Power"=w264) -> (w266:T16)
            n149 = Bundle By Name(cluster=w267, "Output Data Process Image.Contactor Settings(*All Check Out).Station 5"=w266) -> (w265:T2)
          }
          frame 1 {
            n150 = Unbundle By Name(w272) -> ("Output Data Process Image.Contactor Settings(*All Check Out).Station 5"=w274:T16)
            n151 = call "UTILITY Bool to String.vi"("Input Bool"=w270) -> ("Output String"=w269:string)  [unwired: 10 in]
            n152 = Bundle By Name(cluster=w274, "50 Hz Power"=w270) -> (w273:T16)
            n153 = Bundle By Name(cluster=w272, "Output Data Process Image.Contactor Settings(*All Check Out).Station 5"=w273) -> (w271:T2)
          }
          frame 2 {
            n154 = Unbundle By Name(w278) -> ("Output Data Process Image.Contactor Settings(*All Check Out).Station 5"=w280:T16)
            n155 = call "UTILITY Bool to String.vi"("Input Bool"=w276) -> ("Output String"=w275:string)  [unwired: 10 in]
            n156 = Bundle By Name(cluster=w280, "120V Range"=w276) -> (w279:T16)
            n157 = Bundle By Name(cluster=w278, "Output Data Process Image.Contactor Settings(*All Check Out).Station 5"=w279) -> (w277:T2)
          }
          frame 3 {
            n158 = Unbundle By Name(w284) -> ("Output Data Process Image.Contactor Settings(*All Check Out).Station 5"=w286:T16)
            n159 = call "UTILITY Bool to String.vi"("Input Bool"=w282) -> ("Output String"=w281:string)  [unwired: 10 in]
            n160 = Bundle By Name(cluster=w286, "240V Range"=w282) -> (w285:T16)
            n161 = Bundle By Name(cluster=w284, "Output Data Process Image.Contactor Settings(*All Check Out).Station 5"=w285) -> (w283:T2)
          }
          frame 4 {
            n162 = Unbundle By Name(w290) -> ("Output Data Process Image.Contactor Settings(*All Check Out).Station 5"=w292:T16)
            n163 = call "UTILITY Bool to String.vi"("Input Bool"=w288) -> ("Output String"=w287:string)  [unwired: 10 in]
            n164 = Bundle By Name(cluster=w292, "Ground Line"=w288) -> (w291:T16)
            n165 = Bundle By Name(cluster=w290, "Output Data Process Image.Contactor Settings(*All Check Out).Station 5"=w291) -> (w289:T2)
          }
          frame 5 {
            n166 = Unbundle By Name(w296) -> ("Output Data Process Image.Contactor Settings(*All Check Out).Station 5"=w298:T16)
            n167 = call "UTILITY Bool to String.vi"("Input Bool"=w294) -> ("Output String"=w293:string)  [unwired: 10 in]
            n168 = Bundle By Name(cluster=w298, "Ground Neutral"=w294) -> (w297:T16)
            n169 = Bundle By Name(cluster=w296, "Output Data Process Image.Contactor Settings(*All Check Out).Station 5"=w297) -> (w295:T2)
          }
          frame 6 {
            n170 = case shown="True" w301 {
              tunnel: [Wago_Ground_Leakage."1 - Measure GL" ("Ground Leakage") Wago_Ground_Leakage."0 - Normal GL" ("Ground Leakage")] -> w300
              tunnel: ["Measure GL" "Disable GL Measure"] -> w299
              frame False {
              }
              frame True {
              }
            }
            n171 = Unbundle By Name(w303) -> ("Output Data Process Image.Contactor Settings(*All Check Out).Station 5"=w305:T16)
            n172 = Bundle By Name(cluster=w305, "Ground Leakage"=w300) -> (w304:T16)
            n173 = Bundle By Name(cluster=w303, "Output Data Process Image.Contactor Settings(*All Check Out).Station 5"=w304) -> (w302:T2)
          }
          frame 7 {
            n174 = Unbundle By Name(w313) -> ("Output Data Process Image.Contactor Settings(*All Check Out).Station 5"=w315:T16)
            n175 = call "UTILITY Bool to String.vi"("Input Bool"=w311) -> ("Output String"=w310:string)  [unwired: 10 in]
            n176 = Bundle By Name(cluster=w315, "Spare"=w311) -> (w314:T16)
            n177 = Bundle By Name(cluster=w313, "Output Data Process Image.Contactor Settings(*All Check Out).Station 5"=w314) -> (w312:T2)
          }
          frame 8 {
            n178 = Unbundle By Name(w319) -> ("Output Data Process Image.Contactor Settings(*All Check Out).Station 6"=w321:T17)
            n179 = call "UTILITY Bool to String.vi"("Input Bool"=w317) -> ("Output String"=w316:string)  [unwired: 10 in]
            n180 = Bundle By Name(cluster=w321, "60 Hz Power"=w317) -> (w320:T17)
            n181 = Bundle By Name(cluster=w319, "Output Data Process Image.Contactor Settings(*All Check Out).Station 6"=w320) -> (w318:T2)
          }
          frame 9 {
            n182 = Unbundle By Name(w325) -> ("Output Data Process Image.Contactor Settings(*All Check Out).Station 6"=w327:T17)
            n183 = call "UTILITY Bool to String.vi"("Input Bool"=w323) -> ("Output String"=w322:string)  [unwired: 10 in]
            n184 = Bundle By Name(cluster=w327, "50 Hz Power"=w323) -> (w326:T17)
            n185 = Bundle By Name(cluster=w325, "Output Data Process Image.Contactor Settings(*All Check Out).Station 6"=w326) -> (w324:T2)
          }
          frame 10 {
            n186 = Unbundle By Name(w331) -> ("Output Data Process Image.Contactor Settings(*All Check Out).Station 6"=w333:T17)
            n187 = call "UTILITY Bool to String.vi"("Input Bool"=w329) -> ("Output String"=w328:string)  [unwired: 10 in]
            n188 = Bundle By Name(cluster=w333, "120V Range"=w329) -> (w332:T17)
            n189 = Bundle By Name(cluster=w331, "Output Data Process Image.Contactor Settings(*All Check Out).Station 6"=w332) -> (w330:T2)
          }
          frame 11 {
            n190 = Unbundle By Name(w337) -> ("Output Data Process Image.Contactor Settings(*All Check Out).Station 6"=w339:T17)
            n191 = call "UTILITY Bool to String.vi"("Input Bool"=w335) -> ("Output String"=w334:string)  [unwired: 10 in]
            n192 = Bundle By Name(cluster=w339, "240V Range"=w335) -> (w338:T17)
            n193 = Bundle By Name(cluster=w337, "Output Data Process Image.Contactor Settings(*All Check Out).Station 6"=w338) -> (w336:T2)
          }
          frame 12 {
            n194 = Unbundle By Name(w343) -> ("Output Data Process Image.Contactor Settings(*All Check Out).Station 6"=w345:T17)
            n195 = call "UTILITY Bool to String.vi"("Input Bool"=w341) -> ("Output String"=w340:string)  [unwired: 10 in]
            n196 = Bundle By Name(cluster=w345, "Ground Line"=w341) -> (w344:T17)
            n197 = Bundle By Name(cluster=w343, "Output Data Process Image.Contactor Settings(*All Check Out).Station 6"=w344) -> (w342:T2)
          }
          frame 13 {
            n198 = Unbundle By Name(w349) -> ("Output Data Process Image.Contactor Settings(*All Check Out).Station 6"=w351:T17)
            n199 = call "UTILITY Bool to String.vi"("Input Bool"=w347) -> ("Output String"=w346:string)  [unwired: 10 in]
            n200 = Bundle By Name(cluster=w351, "Ground Neutral"=w347) -> (w350:T17)
            n201 = Bundle By Name(cluster=w349, "Output Data Process Image.Contactor Settings(*All Check Out).Station 6"=w350) -> (w348:T2)
          }
          frame 14 {
            n202 = case shown="True" w354 {
              tunnel: [Wago_Ground_Leakage."1 - Measure GL" ("Ground Leakage") Wago_Ground_Leakage."0 - Normal GL" ("Ground Leakage")] -> w353
              tunnel: ["Measure GL" "Disable GL Measure"] -> w352
              frame False {
              }
              frame True {
              }
            }
            n203 = Unbundle By Name(w356) -> ("Output Data Process Image.Contactor Settings(*All Check Out).Station 6"=w358:T17)
            n204 = Bundle By Name(cluster=w358, "Ground Leakage"=w353) -> (w357:T17)
            n205 = Bundle By Name(cluster=w356, "Output Data Process Image.Contactor Settings(*All Check Out).Station 6"=w357) -> (w355:T2)
          }
          frame 15 {
            n206 = Unbundle By Name(w366) -> ("Output Data Process Image.Contactor Settings(*All Check Out).Station 6"=w368:T17)
            n207 = call "UTILITY Bool to String.vi"("Input Bool"=w364) -> ("Output String"=w363:string)  [unwired: 10 in]
            n208 = Bundle By Name(cluster=w368, "Room Pump"=w364) -> (w367:T17)
            n209 = Bundle By Name(cluster=w366, "Output Data Process Image.Contactor Settings(*All Check Out).Station 6"=w367) -> (w365:T2)
          }
        }
      }
      n210 = Build Array(string[] ["60 Hz Power", "50 Hz Power", "120V Range", "240V Range", "Ground Line", "Ground Neutral", "Measure Ground Leakage Current (mA)", "Spare", "60 Hz Power", "50 Hz Power", "120V Range", "240V Range", "Ground Line", "Ground Neutral", "Measure Ground Leakage Current (mA)", "Room Pump"], w252) -> (w255:string[][])
      n211 = Unbundle By Name(w251) -> ("System Send Data"=w250:string[][])
      n212 = Transpose 2D Array(2D array=w255) -> (transposed array=w249:string[][])
      n213 = Build Array (concatenate)(w250, w249) -> (w248:string[][])
      n214 = Bundle By Name(cluster=w251, "System Send Data"=w248) -> (w254:T2)
    }
    frame 519 {
      n215 = for {
        tunnel: w377 -> [w381] mode=indexing
        shift-right: [w380] -> w371
        shift-left: w378 -> [w383]
        tunnel: [w379] -> w373 mode=indexing
        i -> [w382]
        n216 = case shown="1" w382 {
          tunnel: w383 -> [w388 w393 w399 w405 w411 w417 w424 w434 w440 w446 w452 w458 w464 w470 w477 w487]
          tunnel: w381 -> [w385 w391 w397 w403 w409 w415 w422 w432 w438 w444 w450 w456 w462 w468 w475 w485]
          tunnel: [w386 w392 w398 w404 w410 w416 w423 w433 w439 w445 w451 w457 w463 w469 w476 w486] -> w380
          tunnel: [w384 w390 w396 w402 w408 w414 w420 w431 w437 w443 w449 w455 w461 w467 w473 w484] -> w379
          frame 0, Default {
            n217 = Unbundle By Name(w388) -> ("Output Data Process Image.Contactor Settings(*All Check Out).Station 7"=w389:T16)
            n218 = call "UTILITY Bool to String.vi"("Input Bool"=w385) -> ("Output String"=w384:string)  [unwired: 10 in]
            n219 = Bundle By Name(cluster=w389, "60 Hz Power"=w385) -> (w387:T16)
            n220 = Bundle By Name(cluster=w388, "Output Data Process Image.Contactor Settings(*All Check Out).Station 7"=w387) -> (w386:T2)
          }
          frame 1 {
            n221 = Unbundle By Name(w393) -> ("Output Data Process Image.Contactor Settings(*All Check Out).Station 7"=w395:T16)
            n222 = call "UTILITY Bool to String.vi"("Input Bool"=w391) -> ("Output String"=w390:string)  [unwired: 10 in]
            n223 = Bundle By Name(cluster=w395, "50 Hz Power"=w391) -> (w394:T16)
            n224 = Bundle By Name(cluster=w393, "Output Data Process Image.Contactor Settings(*All Check Out).Station 7"=w394) -> (w392:T2)
          }
          frame 2 {
            n225 = Unbundle By Name(w399) -> ("Output Data Process Image.Contactor Settings(*All Check Out).Station 7"=w401:T16)
            n226 = call "UTILITY Bool to String.vi"("Input Bool"=w397) -> ("Output String"=w396:string)  [unwired: 10 in]
            n227 = Bundle By Name(cluster=w401, "120V Range"=w397) -> (w400:T16)
            n228 = Bundle By Name(cluster=w399, "Output Data Process Image.Contactor Settings(*All Check Out).Station 7"=w400) -> (w398:T2)
          }
          frame 3 {
            n229 = Unbundle By Name(w405) -> ("Output Data Process Image.Contactor Settings(*All Check Out).Station 7"=w407:T16)
            n230 = call "UTILITY Bool to String.vi"("Input Bool"=w403) -> ("Output String"=w402:string)  [unwired: 10 in]
            n231 = Bundle By Name(cluster=w407, "240V Range"=w403) -> (w406:T16)
            n232 = Bundle By Name(cluster=w405, "Output Data Process Image.Contactor Settings(*All Check Out).Station 7"=w406) -> (w404:T2)
          }
          frame 4 {
            n233 = Unbundle By Name(w411) -> ("Output Data Process Image.Contactor Settings(*All Check Out).Station 7"=w413:T16)
            n234 = call "UTILITY Bool to String.vi"("Input Bool"=w409) -> ("Output String"=w408:string)  [unwired: 10 in]
            n235 = Bundle By Name(cluster=w413, "Ground Line"=w409) -> (w412:T16)
            n236 = Bundle By Name(cluster=w411, "Output Data Process Image.Contactor Settings(*All Check Out).Station 7"=w412) -> (w410:T2)
          }
          frame 5 {
            n237 = Unbundle By Name(w417) -> ("Output Data Process Image.Contactor Settings(*All Check Out).Station 7"=w419:T16)
            n238 = call "UTILITY Bool to String.vi"("Input Bool"=w415) -> ("Output String"=w414:string)  [unwired: 10 in]
            n239 = Bundle By Name(cluster=w419, "Ground Neutral"=w415) -> (w418:T16)
            n240 = Bundle By Name(cluster=w417, "Output Data Process Image.Contactor Settings(*All Check Out).Station 7"=w418) -> (w416:T2)
          }
          frame 6 {
            n241 = case shown="True" w422 {
              tunnel: [Wago_Ground_Leakage."1 - Measure GL" ("Ground Leakage") Wago_Ground_Leakage."0 - Normal GL" ("Ground Leakage")] -> w421
              tunnel: ["Measure GL" "Disable GL Measure"] -> w420
              frame False {
              }
              frame True {
              }
            }
            n242 = Unbundle By Name(w424) -> ("Output Data Process Image.Contactor Settings(*All Check Out).Station 7"=w426:T16)
            n243 = Bundle By Name(cluster=w426, "Ground Leakage"=w421) -> (w425:T16)
            n244 = Bundle By Name(cluster=w424, "Output Data Process Image.Contactor Settings(*All Check Out).Station 7"=w425) -> (w423:T2)
          }
          frame 7 {
            n245 = Unbundle By Name(w434) -> ("Output Data Process Image.Contactor Settings(*All Check Out).Station 7"=w436:T16)
            n246 = call "UTILITY Bool to String.vi"("Input Bool"=w432) -> ("Output String"=w431:string)  [unwired: 10 in]
            n247 = Bundle By Name(cluster=w436, "Spare"=w432) -> (w435:T16)
            n248 = Bundle By Name(cluster=w434, "Output Data Process Image.Contactor Settings(*All Check Out).Station 7"=w435) -> (w433:T2)
          }
          frame 8 {
            n249 = Unbundle By Name(w440) -> ("Output Data Process Image.Contactor Settings(*All Check Out).Station 8"=w442:T16)
            n250 = call "UTILITY Bool to String.vi"("Input Bool"=w438) -> ("Output String"=w437:string)  [unwired: 10 in]
            n251 = Bundle By Name(cluster=w442, "60 Hz Power"=w438) -> (w441:T16)
            n252 = Bundle By Name(cluster=w440, "Output Data Process Image.Contactor Settings(*All Check Out).Station 8"=w441) -> (w439:T2)
          }
          frame 9 {
            n253 = Unbundle By Name(w446) -> ("Output Data Process Image.Contactor Settings(*All Check Out).Station 8"=w448:T16)
            n254 = call "UTILITY Bool to String.vi"("Input Bool"=w444) -> ("Output String"=w443:string)  [unwired: 10 in]
            n255 = Bundle By Name(cluster=w448, "50 Hz Power"=w444) -> (w447:T16)
            n256 = Bundle By Name(cluster=w446, "Output Data Process Image.Contactor Settings(*All Check Out).Station 8"=w447) -> (w445:T2)
          }
          frame 10 {
            n257 = Unbundle By Name(w452) -> ("Output Data Process Image.Contactor Settings(*All Check Out).Station 8"=w454:T16)
            n258 = call "UTILITY Bool to String.vi"("Input Bool"=w450) -> ("Output String"=w449:string)  [unwired: 10 in]
            n259 = Bundle By Name(cluster=w454, "120V Range"=w450) -> (w453:T16)
            n260 = Bundle By Name(cluster=w452, "Output Data Process Image.Contactor Settings(*All Check Out).Station 8"=w453) -> (w451:T2)
          }
          frame 11 {
            n261 = Unbundle By Name(w458) -> ("Output Data Process Image.Contactor Settings(*All Check Out).Station 8"=w460:T16)
            n262 = call "UTILITY Bool to String.vi"("Input Bool"=w456) -> ("Output String"=w455:string)  [unwired: 10 in]
            n263 = Bundle By Name(cluster=w460, "240V Range"=w456) -> (w459:T16)
            n264 = Bundle By Name(cluster=w458, "Output Data Process Image.Contactor Settings(*All Check Out).Station 8"=w459) -> (w457:T2)
          }
          frame 12 {
            n265 = Unbundle By Name(w464) -> ("Output Data Process Image.Contactor Settings(*All Check Out).Station 8"=w466:T16)
            n266 = call "UTILITY Bool to String.vi"("Input Bool"=w462) -> ("Output String"=w461:string)  [unwired: 10 in]
            n267 = Bundle By Name(cluster=w466, "Ground Line"=w462) -> (w465:T16)
            n268 = Bundle By Name(cluster=w464, "Output Data Process Image.Contactor Settings(*All Check Out).Station 8"=w465) -> (w463:T2)
          }
          frame 13 {
            n269 = Unbundle By Name(w470) -> ("Output Data Process Image.Contactor Settings(*All Check Out).Station 8"=w472:T16)
            n270 = Bundle By Name(cluster=w472, "Ground Neutral"=w468) -> (w471:T16)
            n271 = call "UTILITY Bool to String.vi"("Input Bool"=w468) -> ("Output String"=w467:string)  [unwired: 10 in]
            n272 = Bundle By Name(cluster=w470, "Output Data Process Image.Contactor Settings(*All Check Out).Station 8"=w471) -> (w469:T2)
          }
          frame 14 {
            n273 = case shown="False" w475 {
              tunnel: [Wago_Ground_Leakage."1 - Measure GL" ("Ground Leakage") Wago_Ground_Leakage."0 - Normal GL" ("Ground Leakage")] -> w474
              tunnel: ["Measure GL" "Disable GL Measure"] -> w473
              frame False {
              }
              frame True {
              }
            }
            n274 = Unbundle By Name(w477) -> ("Output Data Process Image.Contactor Settings(*All Check Out).Station 8"=w479:T16)
            n275 = Bundle By Name(cluster=w479, "Ground Leakage"=w474) -> (w478:T16)
            n276 = Bundle By Name(cluster=w477, "Output Data Process Image.Contactor Settings(*All Check Out).Station 8"=w478) -> (w476:T2)
          }
          frame 15 {
            n277 = Unbundle By Name(w487) -> ("Output Data Process Image.Contactor Settings(*All Check Out).Station 8"=w489:T16)
            n278 = call "UTILITY Bool to String.vi"("Input Bool"=w485) -> ("Output String"=w484:string)  [unwired: 10 in]
            n279 = Bundle By Name(cluster=w489, "Spare"=w485) -> (w488:T16)
            n280 = Bundle By Name(cluster=w487, "Output Data Process Image.Contactor Settings(*All Check Out).Station 8"=w488) -> (w486:T2)
          }
        }
      }
      n281 = Build Array(string[] ["60 Hz Power", "50 Hz Power", "120V Range", "240V Range", "Ground Line", "Ground Neutral", "Measure Ground Leakage Current (mA)", "Room OK", "60 Hz Power", "50 Hz Power", "120V Range", "240V Range", "Ground Line", "Ground Neutral", "Measure Ground Leakage Current (mA)", "Fault"], w373) -> (w376:string[][])
      n282 = Transpose 2D Array(2D array=w376) -> (transposed array=w370:string[][])
      n283 = Unbundle By Name(w371) -> ("System Send Data"=w372:string[][])
      n284 = Build Array (concatenate)(w372, w370) -> (w369:string[][])
      n285 = Bundle By Name(cluster=w371, "System Send Data"=w369) -> (w375:T2)
    }
    frame 520 {
      n286 = for {
        tunnel: w498 -> [w502] mode=indexing
        shift-right: [w501] -> w492
        shift-left: w499 -> [w504]
        tunnel: [w500] -> w494 mode=indexing
        i -> [w503]
        n287 = case shown="15" w503 {
          tunnel: w504 -> [w509 w514 w520 w526 w532 w538 w544 w550 w556 w562 w568 w574 w580 w586 w592 w598]
          tunnel: w502 -> [w506 w512 w518 w524 w530 w536 w542 w548 w554 w560 w566 w572 w578 w584 w590 w596]
          tunnel: [w507 w513 w519 w525 w531 w537 w543 w549 w555 w561 w567 w573 w579 w585 w591 w597] -> w501
          tunnel: [w505 w511 w517 w523 w529 w535 w541 w547 w553 w559 w565 w571 w577 w583 w589 w595] -> w500
          frame 0, Default {
            n288 = Unbundle By Name(w509) -> ("Output Data Process Image.Door Output Relays"=w510:T5)
            n289 = call "UTILITY Bool to String.vi"("Input Bool"=w506) -> ("Output String"=w505:string)  [unwired: 10 in]
            n290 = Bundle By Name(cluster=w510, "Station 1 Freezer"=w506) -> (w508:T5)
            n291 = Bundle By Name(cluster=w509, "Output Data Process Image.Door Output Relays"=w508) -> (w507:T2)
          }
          frame 1 {
            n292 = Unbundle By Name(w514) -> ("Output Data Process Image.Door Output Relays"=w516:T5)
            n293 = call "UTILITY Bool to String.vi"("Input Bool"=w512) -> ("Output String"=w511:string)  [unwired: 10 in]
            n294 = Bundle By Name(cluster=w516, "Station 1 Cab"=w512) -> (w515:T5)
            n295 = Bundle By Name(cluster=w514, "Output Data Process Image.Door Output Relays"=w515) -> (w513:T2)
          }
          frame 2 {
            n296 = Unbundle By Name(w520) -> ("Output Data Process Image.Door Output Relays"=w522:T5)
            n297 = call "UTILITY Bool to String.vi"("Input Bool"=w518) -> ("Output String"=w517:string)  [unwired: 10 in]
            n298 = Bundle By Name(cluster=w522, "Station 1 Slide"=w518) -> (w521:T5)
            n299 = Bundle By Name(cluster=w520, "Output Data Process Image.Door Output Relays"=w521) -> (w519:T2)
          }
          frame 3 {
            n300 = Unbundle By Name(w526) -> ("Output Data Process Image.Door Output Relays"=w528:T5)
            n301 = Bundle By Name(cluster=w528, "Station 2 Freezer"=w524) -> (w527:T5)
            n302 = call "UTILITY Bool to String.vi"("Input Bool"=w524) -> ("Output String"=w523:string)  [unwired: 10 in]
            n303 = Bundle By Name(cluster=w526, "Output Data Process Image.Door Output Relays"=w527) -> (w525:T2)
          }
          frame 4 {
            n304 = Unbundle By Name(w532) -> ("Output Data Process Image.Door Output Relays"=w534:T5)
            n305 = Bundle By Name(cluster=w534, "Station 2 Cab"=w530) -> (w533:T5)
            n306 = call "UTILITY Bool to String.vi"("Input Bool"=w530) -> ("Output String"=w529:string)  [unwired: 10 in]
            n307 = Bundle By Name(cluster=w532, "Output Data Process Image.Door Output Relays"=w533) -> (w531:T2)
          }
          frame 5 {
            n308 = Unbundle By Name(w538) -> ("Output Data Process Image.Door Output Relays"=w540:T5)
            n309 = Bundle By Name(cluster=w540, "Station 2 Slide"=w536) -> (w539:T5)
            n310 = call "UTILITY Bool to String.vi"("Input Bool"=w536) -> ("Output String"=w535:string)  [unwired: 10 in]
            n311 = Bundle By Name(cluster=w538, "Output Data Process Image.Door Output Relays"=w539) -> (w537:T2)
          }
          frame 6 {
            n312 = Unbundle By Name(w544) -> ("Output Data Process Image.Door Output Relays"=w546:T5)
            n313 = call "UTILITY Bool to String.vi"("Input Bool"=w542) -> ("Output String"=w541:string)  [unwired: 10 in]
            n314 = Bundle By Name(cluster=w546, "Station 3 Freezer"=w542) -> (w545:T5)
            n315 = Bundle By Name(cluster=w544, "Output Data Process Image.Door Output Relays"=w545) -> (w543:T2)
          }
          frame 7 {
            n316 = Unbundle By Name(w550) -> ("Output Data Process Image.Door Output Relays"=w552:T5)
            n317 = call "UTILITY Bool to String.vi"("Input Bool"=w548) -> ("Output String"=w547:string)  [unwired: 10 in]
            n318 = Bundle By Name(cluster=w552, "Station 3 Cab"=w548) -> (w551:T5)
            n319 = Bundle By Name(cluster=w550, "Output Data Process Image.Door Output Relays"=w551) -> (w549:T2)
          }
          frame 8 {
            n320 = Unbundle By Name(w556) -> ("Output Data Process Image.Door Output Relays"=w558:T5)
            n321 = call "UTILITY Bool to String.vi"("Input Bool"=w554) -> ("Output String"=w553:string)  [unwired: 10 in]
            n322 = Bundle By Name(cluster=w558, "Station 3 Slide"=w554) -> (w557:T5)
            n323 = Bundle By Name(cluster=w556, "Output Data Process Image.Door Output Relays"=w557) -> (w555:T2)
          }
          frame 9 {
            n324 = Unbundle By Name(w562) -> ("Output Data Process Image.Door Output Relays"=w564:T5)
            n325 = Bundle By Name(cluster=w564, "Station 4 Freezer"=w560) -> (w563:T5)
            n326 = call "UTILITY Bool to String.vi"("Input Bool"=w560) -> ("Output String"=w559:string)  [unwired: 10 in]
            n327 = Bundle By Name(cluster=w562, "Output Data Process Image.Door Output Relays"=w563) -> (w561:T2)
          }
          frame 10 {
            n328 = Unbundle By Name(w568) -> ("Output Data Process Image.Door Output Relays"=w570:T5)
            n329 = call "UTILITY Bool to String.vi"("Input Bool"=w566) -> ("Output String"=w565:string)  [unwired: 10 in]
            n330 = Bundle By Name(cluster=w570, "Station 4 Cab"=w566) -> (w569:T5)
            n331 = Bundle By Name(cluster=w568, "Output Data Process Image.Door Output Relays"=w569) -> (w567:T2)
          }
          frame 11 {
            n332 = Unbundle By Name(w574) -> ("Output Data Process Image.Door Output Relays"=w576:T5)
            n333 = call "UTILITY Bool to String.vi"("Input Bool"=w572) -> ("Output String"=w571:string)  [unwired: 10 in]
            n334 = Bundle By Name(cluster=w576, "Station 4 Slide"=w572) -> (w575:T5)
            n335 = Bundle By Name(cluster=w574, "Output Data Process Image.Door Output Relays"=w575) -> (w573:T2)
          }
          frame 12 {
            n336 = Unbundle By Name(w580) -> ("Output Data Process Image.Door Output Relays"=w582:T5)
            n337 = call "UTILITY Bool to String.vi"("Input Bool"=w578) -> ("Output String"=w577:string)  [unwired: 10 in]
            n338 = Bundle By Name(cluster=w582, "Station 5 Freezer"=w578) -> (w581:T5)
            n339 = Bundle By Name(cluster=w580, "Output Data Process Image.Door Output Relays"=w581) -> (w579:T2)
          }
          frame 13 {
            n340 = Unbundle By Name(w586) -> ("Output Data Process Image.Door Output Relays"=w588:T5)
            n341 = Bundle By Name(cluster=w588, "Station 5 Cab"=w584) -> (w587:T5)
            n342 = call "UTILITY Bool to String.vi"("Input Bool"=w584) -> ("Output String"=w583:string)  [unwired: 10 in]
            n343 = Bundle By Name(cluster=w586, "Output Data Process Image.Door Output Relays"=w587) -> (w585:T2)
          }
          frame 14 {
            n344 = Unbundle By Name(w592) -> ("Output Data Process Image.Door Output Relays"=w594:T5)
            n345 = call "UTILITY Bool to String.vi"("Input Bool"=w590) -> ("Output String"=w589:string)  [unwired: 10 in]
            n346 = Bundle By Name(cluster=w594, "Station 5 Slide"=w590) -> (w593:T5)
            n347 = Bundle By Name(cluster=w592, "Output Data Process Image.Door Output Relays"=w593) -> (w591:T2)
          }
          frame 15 {
            n348 = Unbundle By Name(w598) -> ("Output Data Process Image.Door Output Relays"=w600:T5)
            n349 = Bundle By Name(cluster=w600, "Station 6 Freezer"=w596) -> (w599:T5)
            n350 = call "UTILITY Bool to String.vi"("Input Bool"=w596) -> ("Output String"=w595:string)  [unwired: 10 in]
            n351 = Bundle By Name(cluster=w598, "Output Data Process Image.Door Output Relays"=w599) -> (w597:T2)
          }
        }
      }
      n352 = Build Array(string[] ["Station 1 Freezer", "Station 1 Cab", "Station 1 Slide", "Station 2 Freezer", "Station 2 Cab", "Station 2 Slide", "Station 3 Freezer", "Station 3 Cab", "Station 3 Slide", "Station 4 Freezer", "Station 4 Cab", "Station 4 Slide", "Station 5 Freezer", "Station 5 Cab", "Station 5 Slide", "Station 6 Freezer"], w494) -> (w497:string[][])
      n353 = Transpose 2D Array(2D array=w497) -> (transposed array=w491:string[][])
      n354 = Unbundle By Name(w492) -> ("System Send Data"=w493:string[][])
      n355 = Build Array (concatenate)(w493, w491) -> (w490:string[][])
      n356 = Bundle By Name(cluster=w492, "System Send Data"=w490) -> (w496:T2)
    }
    frame 521 {
      n357 = for {
        tunnel: w609 -> [w613] mode=indexing
        shift-right: [w612] -> w603
        shift-left: w610 -> [w615]
        tunnel: [w611] -> w605 mode=indexing
        i -> [w614]
        n358 = case shown="15" w614 {
          tunnel: w615 -> [w620 w625 w631 w637 w643 w649 w655 w661 w667 w673 w679 w685 w691 w697 w703 w709]
          tunnel: w613 -> [w617 w623 w629 w635 w641 w647 w653 w659 w665 w671 w677 w683 w689 w695 w701 w707]
          tunnel: [w618 w624 w630 w636 w642 w648 w654 w660 w666 w672 w678 w684 w690 w696 w702 w708] -> w612
          tunnel: [w616 w622 w628 w634 w640 w646 w652 w658 w664 w670 w676 w682 w688 w694 w700 w706] -> w611
          frame 0, Default {
            n359 = Unbundle By Name(w620) -> ("Output Data Process Image.Door Output Relays"=w621:T5)
            n360 = Bundle By Name(cluster=w621, "Station 6 Cab"=w617) -> (w619:T5)
            n361 = call "UTILITY Bool to String.vi"("Input Bool"=w617) -> ("Output String"=w616:string)  [unwired: 10 in]
            n362 = Bundle By Name(cluster=w620, "Output Data Process Image.Door Output Relays"=w619) -> (w618:T2)
          }
          frame 1 {
            n363 = Unbundle By Name(w625) -> ("Output Data Process Image.Door Output Relays"=w627:T5)
            n364 = Bundle By Name(cluster=w627, "Station 6 Slide"=w623) -> (w626:T5)
            n365 = call "UTILITY Bool to String.vi"("Input Bool"=w623) -> ("Output String"=w622:string)  [unwired: 10 in]
            n366 = Bundle By Name(cluster=w625, "Output Data Process Image.Door Output Relays"=w626) -> (w624:T2)
          }
          frame 2 {
            n367 = Unbundle By Name(w631) -> ("Output Data Process Image.Door Output Relays"=w633:T5)
            n368 = Bundle By Name(cluster=w633, "Station 7 Freezer"=w629) -> (w632:T5)
            n369 = call "UTILITY Bool to String.vi"("Input Bool"=w629) -> ("Output String"=w628:string)  [unwired: 10 in]
            n370 = Bundle By Name(cluster=w631, "Output Data Process Image.Door Output Relays"=w632) -> (w630:T2)
          }
          frame 3 {
            n371 = Unbundle By Name(w637) -> ("Output Data Process Image.Door Output Relays"=w639:T5)
            n372 = Bundle By Name(cluster=w639, "Station 7 Cab"=w635) -> (w638:T5)
            n373 = call "UTILITY Bool to String.vi"("Input Bool"=w635) -> ("Output String"=w634:string)  [unwired: 10 in]
            n374 = Bundle By Name(cluster=w637, "Output Data Process Image.Door Output Relays"=w638) -> (w636:T2)
          }
          frame 4 {
            n375 = Unbundle By Name(w643) -> ("Output Data Process Image.Door Output Relays"=w645:T5)
            n376 = Bundle By Name(cluster=w645, "Station 7 Slide"=w641) -> (w644:T5)
            n377 = call "UTILITY Bool to String.vi"("Input Bool"=w641) -> ("Output String"=w640:string)  [unwired: 10 in]
            n378 = Bundle By Name(cluster=w643, "Output Data Process Image.Door Output Relays"=w644) -> (w642:T2)
          }
          frame 5 {
            n379 = Unbundle By Name(w649) -> ("Output Data Process Image.Door Output Relays"=w651:T5)
            n380 = Bundle By Name(cluster=w651, "Station 8 Freezer"=w647) -> (w650:T5)
            n381 = call "UTILITY Bool to String.vi"("Input Bool"=w647) -> ("Output String"=w646:string)  [unwired: 10 in]
            n382 = Bundle By Name(cluster=w649, "Output Data Process Image.Door Output Relays"=w650) -> (w648:T2)
          }
          frame 6 {
            n383 = Unbundle By Name(w655) -> ("Output Data Process Image.Door Output Relays"=w657:T5)
            n384 = Bundle By Name(cluster=w657, "Station 8 Cab"=w653) -> (w656:T5)
            n385 = call "UTILITY Bool to String.vi"("Input Bool"=w653) -> ("Output String"=w652:string)  [unwired: 10 in]
            n386 = Bundle By Name(cluster=w655, "Output Data Process Image.Door Output Relays"=w656) -> (w654:T2)
          }
          frame 7 {
            n387 = Unbundle By Name(w661) -> ("Output Data Process Image.Door Output Relays"=w663:T5)
            n388 = Bundle By Name(cluster=w663, "Station 8 Slide"=w659) -> (w662:T5)
            n389 = call "UTILITY Bool to String.vi"("Input Bool"=w659) -> ("Output String"=w658:string)  [unwired: 10 in]
            n390 = Bundle By Name(cluster=w661, "Output Data Process Image.Door Output Relays"=w662) -> (w660:T2)
          }
          frame 8 {
            n391 = Unbundle By Name(w667) -> ("Output Data Process Image.Variac Output(*All Check Out)"=w669:T18)
            n392 = Bundle By Name(cluster=w669, "Station 1 Volt Increase"=w665) -> (w668:T18)
            n393 = call "UTILITY Bool to String.vi"("Input Bool"=w665) -> ("Output String"=w664:string)  [unwired: 10 in]
            n394 = Bundle By Name(cluster=w667, "Output Data Process Image.Variac Output(*All Check Out)"=w668) -> (w666:T2)
          }
          frame 9 {
            n395 = Unbundle By Name(w673) -> ("Output Data Process Image.Variac Output(*All Check Out)"=w675:T18)
            n396 = Bundle By Name(cluster=w675, "Station 1 Volt Decrease"=w671) -> (w674:T18)
            n397 = call "UTILITY Bool to String.vi"("Input Bool"=w671) -> ("Output String"=w670:string)  [unwired: 10 in]
            n398 = Bundle By Name(cluster=w673, "Output Data Process Image.Variac Output(*All Check Out)"=w674) -> (w672:T2)
          }
          frame 10 {
            n399 = Unbundle By Name(w679) -> ("Output Data Process Image.Variac Output(*All Check Out)"=w681:T18)
            n400 = Bundle By Name(cluster=w681, "Station 2 Volt Increase"=w677) -> (w680:T18)
            n401 = call "UTILITY Bool to String.vi"("Input Bool"=w677) -> ("Output String"=w676:string)  [unwired: 10 in]
            n402 = Bundle By Name(cluster=w679, "Output Data Process Image.Variac Output(*All Check Out)"=w680) -> (w678:T2)
          }
          frame 11 {
            n403 = Unbundle By Name(w685) -> ("Output Data Process Image.Variac Output(*All Check Out)"=w687:T18)
            n404 = Bundle By Name(cluster=w687, "Station 2 Volt Decrease"=w683) -> (w686:T18)
            n405 = call "UTILITY Bool to String.vi"("Input Bool"=w683) -> ("Output String"=w682:string)  [unwired: 10 in]
            n406 = Bundle By Name(cluster=w685, "Output Data Process Image.Variac Output(*All Check Out)"=w686) -> (w684:T2)
          }
          frame 12 {
            n407 = Unbundle By Name(w691) -> ("Output Data Process Image.Variac Output(*All Check Out)"=w693:T18)
            n408 = Bundle By Name(cluster=w693, "Station 3 Volt Increase"=w689) -> (w692:T18)
            n409 = call "UTILITY Bool to String.vi"("Input Bool"=w689) -> ("Output String"=w688:string)  [unwired: 10 in]
            n410 = Bundle By Name(cluster=w691, "Output Data Process Image.Variac Output(*All Check Out)"=w692) -> (w690:T2)
          }
          frame 13 {
            n411 = Unbundle By Name(w697) -> ("Output Data Process Image.Variac Output(*All Check Out)"=w699:T18)
            n412 = Bundle By Name(cluster=w699, "Station 3 Volt Decrease"=w695) -> (w698:T18)
            n413 = call "UTILITY Bool to String.vi"("Input Bool"=w695) -> ("Output String"=w694:string)  [unwired: 10 in]
            n414 = Bundle By Name(cluster=w697, "Output Data Process Image.Variac Output(*All Check Out)"=w698) -> (w696:T2)
          }
          frame 14 {
            n415 = Unbundle By Name(w703) -> ("Output Data Process Image.Variac Output(*All Check Out)"=w705:T18)
            n416 = Bundle By Name(cluster=w705, "Station 4 Volt Increase"=w701) -> (w704:T18)
            n417 = call "UTILITY Bool to String.vi"("Input Bool"=w701) -> ("Output String"=w700:string)  [unwired: 10 in]
            n418 = Bundle By Name(cluster=w703, "Output Data Process Image.Variac Output(*All Check Out)"=w704) -> (w702:T2)
          }
          frame 15 {
            n419 = Unbundle By Name(w709) -> ("Output Data Process Image.Variac Output(*All Check Out)"=w711:T18)
            n420 = Bundle By Name(cluster=w711, "Station 4 Volt Decrease"=w707) -> (w710:T18)
            n421 = call "UTILITY Bool to String.vi"("Input Bool"=w707) -> ("Output String"=w706:string)  [unwired: 10 in]
            n422 = Bundle By Name(cluster=w709, "Output Data Process Image.Variac Output(*All Check Out)"=w710) -> (w708:T2)
          }
        }
      }
      n423 = Unbundle By Name(w603) -> ("System Send Data"=w604:string[][])
      n424 = Build Array(string[] ["Station 6 Cab", "Station 6 Slide", "Station 7 Freezer", "Station 7 Cab", "Station 7 Slide", "Station 8 Freezer", "Station 8 Cab", "Station 8 Slide", "Station 1 Volt Increase", "Station 1 Volt Decrease", "Station 2 Volt Increase", "Station 2 Volt Decrease", "Station 3 Volt Increase", "Station 3 Volt Decrease", "Station 4 Volt Increase", "Station 4 Volt Decrease"], w605) -> (w608:string[][])
      n425 = Transpose 2D Array(2D array=w608) -> (transposed array=w602:string[][])
      n426 = Build Array (concatenate)(w604, w602) -> (w601:string[][])
      n427 = Bundle By Name(cluster=w603, "System Send Data"=w601) -> (w607:T2)
    }
    frame 522 {
      n428 = for {
        N: 8 -> [_]
        tunnel: w721 -> [w725] mode=indexing
        shift-right: [w724] -> w714
        shift-left: w722 -> [w727]
        tunnel: [w723] -> w716 mode=indexing
        i -> [w726]
        n429 = case shown="7" w726 {
          tunnel: w727 -> [w732 w737 w743 w749 w755 w761 w767 w773]
          tunnel: w725 -> [w729 w735 w741 w747 w753 w759 w765 w771]
          tunnel: [w730 w736 w742 w748 w754 w760 w766 w772] -> w724
          tunnel: [w728 w734 w740 w746 w752 w758 w764 w770] -> w723
          frame 0, Default {
            n430 = Unbundle By Name(w732) -> ("Output Data Process Image.Variac Output(*All Check Out)"=w733:T18)
            n431 = Bundle By Name(cluster=w733, "Station 5 Volt Increase"=w729) -> (w731:T18)
            n432 = call "UTILITY Bool to String.vi"("Input Bool"=w729) -> ("Output String"=w728:string)  [unwired: 10 in]
            n433 = Bundle By Name(cluster=w732, "Output Data Process Image.Variac Output(*All Check Out)"=w731) -> (w730:T2)
          }
          frame 1 {
            n434 = Unbundle By Name(w737) -> ("Output Data Process Image.Variac Output(*All Check Out)"=w739:T18)
            n435 = Bundle By Name(cluster=w739, "Station 5 Volt Decrease"=w735) -> (w738:T18)
            n436 = call "UTILITY Bool to String.vi"("Input Bool"=w735) -> ("Output String"=w734:string)  [unwired: 10 in]
            n437 = Bundle By Name(cluster=w737, "Output Data Process Image.Variac Output(*All Check Out)"=w738) -> (w736:T2)
          }
          frame 2 {
            n438 = Unbundle By Name(w743) -> ("Output Data Process Image.Variac Output(*All Check Out)"=w745:T18)
            n439 = Bundle By Name(cluster=w745, "Station 6 Volt Increase"=w741) -> (w744:T18)
            n440 = call "UTILITY Bool to String.vi"("Input Bool"=w741) -> ("Output String"=w740:string)  [unwired: 10 in]
            n441 = Bundle By Name(cluster=w743, "Output Data Process Image.Variac Output(*All Check Out)"=w744) -> (w742:T2)
          }
          frame 3 {
            n442 = Unbundle By Name(w749) -> ("Output Data Process Image.Variac Output(*All Check Out)"=w751:T18)
            n443 = Bundle By Name(cluster=w751, "Station 6 Volt Decrease"=w747) -> (w750:T18)
            n444 = call "UTILITY Bool to String.vi"("Input Bool"=w747) -> ("Output String"=w746:string)  [unwired: 10 in]
            n445 = Bundle By Name(cluster=w749, "Output Data Process Image.Variac Output(*All Check Out)"=w750) -> (w748:T2)
          }
          frame 4 {
            n446 = Unbundle By Name(w755) -> ("Output Data Process Image.Variac Output(*All Check Out)"=w757:T18)
            n447 = Bundle By Name(cluster=w757, "Station 7 Volt Increase"=w753) -> (w756:T18)
            n448 = call "UTILITY Bool to String.vi"("Input Bool"=w753) -> ("Output String"=w752:string)  [unwired: 10 in]
            n449 = Bundle By Name(cluster=w755, "Output Data Process Image.Variac Output(*All Check Out)"=w756) -> (w754:T2)
          }
          frame 5 {
            n450 = Unbundle By Name(w761) -> ("Output Data Process Image.Variac Output(*All Check Out)"=w763:T18)
            n451 = Bundle By Name(cluster=w763, "Station 7 Volt Decrease"=w759) -> (w762:T18)
            n452 = call "UTILITY Bool to String.vi"("Input Bool"=w759) -> ("Output String"=w758:string)  [unwired: 10 in]
            n453 = Bundle By Name(cluster=w761, "Output Data Process Image.Variac Output(*All Check Out)"=w762) -> (w760:T2)
          }
          frame 6 {
            n454 = Unbundle By Name(w767) -> ("Output Data Process Image.Variac Output(*All Check Out)"=w769:T18)
            n455 = Bundle By Name(cluster=w769, "Station 8 Volt Increase"=w765) -> (w768:T18)
            n456 = call "UTILITY Bool to String.vi"("Input Bool"=w765) -> ("Output String"=w764:string)  [unwired: 10 in]
            n457 = Bundle By Name(cluster=w767, "Output Data Process Image.Variac Output(*All Check Out)"=w768) -> (w766:T2)
          }
          frame 7 {
            n458 = Unbundle By Name(w773) -> ("Output Data Process Image.Variac Output(*All Check Out)"=w775:T18)
            n459 = Bundle By Name(cluster=w775, "Station 8 Volt Decrease"=w771) -> (w774:T18)
            n460 = call "UTILITY Bool to String.vi"("Input Bool"=w771) -> ("Output String"=w770:string)  [unwired: 10 in]
            n461 = Bundle By Name(cluster=w773, "Output Data Process Image.Variac Output(*All Check Out)"=w774) -> (w772:T2)
          }
        }
      }
      n462 = Build Array(string[] ["Station 5 Volt Increase", "Station 5 Volt Decrease", "Station 6 Volt Increase", "Station 6 Volt Decrease", "Station 7 Volt Increase", "Station 7 Volt Decrease", "Station 8 Volt Increase", "Station 8 Volt Decrease"], w716) -> (w719:string[][])
      n463 = Transpose 2D Array(2D array=w719) -> (transposed array=w713:string[][])
      n464 = Unbundle By Name(w714) -> ("System Send Data"=w715:string[][])
      n465 = Build Array (concatenate)(w715, w713) -> (w712:string[][])
      n466 = Bundle By Name(cluster=w714, "System Send Data"=w712) -> (w718:T2)
    }
  }
  "Wago Data Input out" <- w3
  "Error Out" <- "Error In"
